vi "RL Connect.vi"() -> ()   [LabVIEW 2019]
uses:
  C:/Users/wego/Documents/GitHub/Ycar/LabVIEW/Gmap/dll/GMap.NET.WindowsForms.dll
  Gmap/dll/GMap.NET.WindowsForms.dll
  Ctrl/ublox-ui_main.ctl
  Ctrl/gnss_config-2.ctl
  Ctrl/Ntrip_Account_db.ctl
  Ctrl/Ntrip error-leds.ctl
  Ctrl/cmd_common.ctl
  Ctrl/cmd_ini-add-read.ctl
  Ctrl/cmd_ini-RW.ctl
  Ctrl/GNSS-Ntrip ref.ctl
  Gmap/gmap_fgv-cmd.ctl
  Ctrl/GNSS-Ntrip config.ctl
  Ctrl/error_state-val.ctl
panel:
  out "Version String":string
  in  "Ntrip connect":bool
  out "status":T1={"GNSS Serial"=0, "NMEA val"=0, "Send Serial"=0, "Ntrip TCP"=0, "RTCM val"=0, "GMAP"=0, "TBD1"=2, "TBD2"=2, "TBD3"=2}
  in  "Send-Serial Start-Stop":bool
  in  "GNSS Start-Stop":bool
  in  "stop":bool
  in  "gmap center":bool
  in  "Gmap Lon":dbl format="%.7f"
  in  "Gmap Lat":dbl format="%.7f"
  in  "GMapControl":refnum<k24>(container)
  out "GNSS time":string
  out "Ntrip conn":bool
  out "NMEA val":bool
  in  "main tap":T2(tab)
  out "TM\nptn":u32(slide) scale=0.0..200.0
  out "Sea Level":dbl
  out "N of Satellites":i32
  out "TM graph":T3(graph)=[{"TM array"=[{"Y(E)"=195478.83340938148, "X(N)"=532749.6315443226}, {"Y(E)"=195478.83340938148, "X(N)"=532749.6315443226}, {"Y(E)"=195478.83340938148, "X(N)"=532749.6315443226}, {"Y(E)"=195478.83340938148, "X(N)"=532749.6315443226}, {"Y(E)"=195478.83340938148, "X(N)"=532749.6315443226}, {"Y(E)"=195478.83340938148, "X(N)"=532749.6315443226}, {"Y(E)"=195478.83340938148, "X(N)"=532749.6315443226}, {"Y(E)"=195478.83340938148, "X(N)"=532749.6315443226}, {"Y(E)"=195478.83340938148, "X(N)"=532749.6315443226}, {"Y(E)"=195478.83340938148, "X(N)"=532749.6315443226}, {"Y(E)"=195478.80387262133, "X(N)"=532749.5945652778}, {"Y(E)"=195478.80387262133, "X(N)"=532749.5945652778}, {"Y(E)"=195478.80387262133, "X(N)"=532749.5945652778}, {"Y(E)"=195478.80387262133, "X(N)"=532749.5945652778}, {"Y(E)"=195478.80387262133, "X(N)"=532749.5945652778}, {"Y(E)"=195478.80387262133, "X(N)"=532749.5945652778}, {"Y(E)"=195478.80387262133, "X(N)"=532749.5945652778}, {"Y(E)"=195478.80387262133, "X(N)"=532749.5945652778}, {"Y(E)"=195478.80387262133, "X(N)"=532749.5945652778}, {"Y(E)"=195478.80387262133, "X(N)"=532749.5945652778}, {"Y(E)"=195478.80387262133, "X(N)"=532749.5945652778}, {"Y(E)"=195478.80387262133, "X(N)"=532749.5945652778}, {"Y(E)"=195478.80387262133, "X(N)"=532749.5945652778}, {"Y(E)"=195478.86283602339, "X(N)"=532749.4650507653}, {"Y(E)"=195478.86283602339, "X(N)"=532749.4650507653}, {"Y(E)"=195478.86283602339, "X(N)"=532749.4650507653}, {"Y(E)"=195478.86283602339, "X(N)"=532749.4650507653}, {"Y(E)"=195478.86283602339, "X(N)"=532749.4650507653}, {"Y(E)"=195478.86283602339, "X(N)"=532749.4650507653}, {"Y(E)"=195478.86283602339, "X(N)"=532749.4650507653}, {"Y(E)"=195478.86283602339, "X(N)"=532749.4650507653}, {"Y(E)"=195478.86283602339, "X(N)"=532749.4650507653}, {"Y(E)"=195478.86283602339, "X(N)"=532749.4650507653}, {"Y(E)"=195478.86283602339, "X(N)"=532749.4650507653}, {"Y(E)"=195478.86283602339, "X(N)"=532749.4650507653}, {"Y(E)"=195478.86283602339, "X(N)"=532749.4650507653}, {"Y(E)"=195478.8185809412, "X(N)"=532749.5020697443}, {"Y(E)"=195478.8185809412, "X(N)"=532749.5020697443}, {"Y(E)"=195478.8185809412, "X(N)"=532749.5020697443}, {"Y(E)"=195478.8185809412, "X(N)"=532749.5020697443}, {"Y(E)"=195478.8185809412, "X(N)"=532749.5020697443}, {"Y(E)"=195478.8185809412, "X(N)"=532749.5020697443}, {"Y(E)"=195478.8185809412, "X(N)"=532749.5020697443}, {"Y(E)"=195478.8185809412, "X(N)"=532749.5020697443}, {"Y(E)"=195478.8185809412, "X(N)"=532749.5020697443}, {"Y(E)"=195478.8185809412, "X(N)"=532749.5020697443}, {"Y(E)"=195478.8185809412, "X(N)"=532749.5020697443}, {"Y(E)"=195478.8185809412, "X(N)"=532749.5020697443}, {"Y(E)"=195478.8185809412, "X(N)"=532749.5020697443}, {"Y(E)"=195478.8333493192, "X(N)"=532749.5205592669}, {"Y(E)"=195478.8333493192, "X(N)"=532749.5205592669}, {"Y(E)"=195478.8333493192, "X(N)"=532749.5205592669}, {"Y(E)"=195478.8333493192, "X(N)"=532749.5205592669}, {"Y(E)"=195478.8333493192, "X(N)"=532749.5205592669}, {"Y(E)"=195478.8333493192, "X(N)"=532749.5205592669}, {"Y(E)"=195478.8333493192, "X(N)"=532749.5205592669}, {"Y(E)"=195478.8333493192, "X(N)"=532749.5205592669}, {"Y(E)"=195478.8333493192, "X(N)"=532749.5205592669}, {"Y(E)"=195478.8333493192, "X(N)"=532749.5205592669}, {"Y(E)"=195478.8333493192, "X(N)"=532749.5205592669}, {"Y(E)"=195478.8333493192, "X(N)"=532749.5205592669}, {"Y(E)"=195478.81854089958, "X(N)"=532749.4280797082}, {"Y(E)"=195478.81854089958, "X(N)"=532749.4280797082}, {"Y(E)"=195478.81854089958, "X(N)"=532749.4280797082}, {"Y(E)"=195478.81854089958, "X(N)"=532749.4280797082}, {"Y(E)"=195478.81854089958, "X(N)"=532749.4280797082}, {"Y(E)"=195478.81854089958, "X(N)"=532749.4280797082}, {"Y(E)"=195478.81854089958, "X(N)"=532749.4280797082}, {"Y(E)"=195478.81854089958, "X(N)"=532749.4280797082}, {"Y(E)"=195478.81854089958, "X(N)"=532749.4280797082}, {"Y(E)"=195478.81854089958, "X(N)"=532749.4280797082}, {"Y(E)"=195478.81854089958, "X(N)"=532749.4280797082}, {"Y(E)"=195478.81854089958, "X(N)"=532749.4280797082}, {"Y(E)"=195478.81854089958, "X(N)"=532749.4280797082}, {"Y(E)"=195478.8332592258, "X(N)"=532749.3540816847}, {"Y(E)"=195478.8332592258, "X(N)"=532749.3540816847}, {"Y(E)"=195478.8332592258, "X(N)"=532749.3540816847}, {"Y(E)"=195478.8332592258, "X(N)"=532749.3540816847}, {"Y(E)"=195478.8332592258, "X(N)"=532749.3540816847}, {"Y(E)"=195478.8332592258, "X(N)"=532749.3540816847}, {"Y(E)"=195478.8332592258, "X(N)"=532749.3540816847}, {"Y(E)"=195478.8332592258, "X(N)"=532749.3540816847}, {"Y(E)"=195478.8332592258, "X(N)"=532749.3540816847}, {"Y(E)"=195478.8332592258, "X(N)"=532749.3540816847}, {"Y(E)"=195478.8332592258, "X(N)"=532749.3540816847}, {"Y(E)"=195478.8332592258, "X(N)"=532749.3540816847}, {"Y(E)"=195478.8332592258, "X(N)"=532749.3540816847}, {"Y(E)"=195478.61200383154, "X(N)"=532749.5761715989}, {"Y(E)"=195478.61200383154, "X(N)"=532749.5761715989}, {"Y(E)"=195478.61200383154, "X(N)"=532749.5761715989}, {"Y(E)"=195478.61200383154, "X(N)"=532749.5761715989}, {"Y(E)"=195478.61200383154, "X(N)"=532749.5761715989}, {"Y(E)"=195478.61200383154, "X(N)"=532749.5761715989}, {"Y(E)"=195478.61200383154, "X(N)"=532749.5761715989}, {"Y(E)"=195478.61200383154, "X(N)"=532749.5761715989}, {"Y(E)"=195478.61200383154, "X(N)"=532749.5761715989}, {"Y(E)"=195478.61200383154, "X(N)"=532749.5761715989}, {"Y(E)"=195478.61200383154, "X(N)"=532749.5761715989}, {"Y(E)"=195478.61200383154, "X(N)"=532749.5761715989}, {"Y(E)"=195478.61200383154, "X(N)"=532749.5761715989}, {"Y(E)"=195478.61197379892, "X(N)"=532749.5206790727}, {"Y(E)"=195478.61197379892, "X(N)"=532749.5206790727}, {"Y(E)"=195478.61197379892, "X(N)"=532749.5206790727}, {"Y(E)"=195478.61197379892, "X(N)"=532749.5206790727}, {"Y(E)"=195478.61197379892, "X(N)"=532749.5206790727}, {"Y(E)"=195478.61197379892, "X(N)"=532749.5206790727}, {"Y(E)"=195478.61197379892, "X(N)"=532749.5206790727}, {"Y(E)"=195478.61197379892, "X(N)"=532749.5206790727}, {"Y(E)"=195478.61197379892, "X(N)"=532749.5206790727}, {"Y(E)"=195478.61197379892, "X(N)"=532749.5206790727}, {"Y(E)"=195478.61197379892, "X(N)"=532749.5206790727}, {"Y(E)"=195478.61197379892, "X(N)"=532749.5206790727}, {"Y(E)"=195478.61197379892, "X(N)"=532749.5206790727}, {"Y(E)"=195478.64144048005, "X(N)"=532749.4281755526}, {"Y(E)"=195478.64144048005, "X(N)"=532749.4281755526}, {"Y(E)"=195478.64144048005, "X(N)"=532749.4281755526}, {"Y(E)"=195478.64144048005, "X(N)"=532749.4281755526}, {"Y(E)"=195478.64144048005, "X(N)"=532749.4281755526}, {"Y(E)"=195478.64144048005, "X(N)"=532749.4281755526}, {"Y(E)"=195478.64144048005, "X(N)"=532749.4281755526}, {"Y(E)"=195478.64144048005, "X(N)"=532749.4281755526}, {"Y(E)"=195478.64144048005, "X(N)"=532749.4281755526}, {"Y(E)"=195478.64144048005, "X(N)"=532749.4281755526}, {"Y(E)"=195478.64144048005, "X(N)"=532749.4281755526}, {"Y(E)"=195478.64144048005, "X(N)"=532749.4281755526}, {"Y(E)"=195478.64144048005, "X(N)"=532749.4281755526}, {"Y(E)"=195478.56754852948, "X(N)"=532749.2432403986}, {"Y(E)"=195478.56754852948, "X(N)"=532749.2432403986}, {"Y(E)"=195478.56754852948, "X(N)"=532749.2432403986}, {"Y(E)"=195478.56754852948, "X(N)"=532749.2432403986}, {"Y(E)"=195478.56754852948, "X(N)"=532749.2432403986}, {"Y(E)"=195478.56754852948, "X(N)"=532749.2432403986}, {"Y(E)"=195478.56754852948, "X(N)"=532749.2432403986}, {"Y(E)"=195478.56754852948, "X(N)"=532749.2432403986}, {"Y(E)"=195478.56754852948, "X(N)"=532749.2432403986}, {"Y(E)"=195478.56754852948, "X(N)"=532749.2432403986}, {"Y(E)"=195478.56754852948, "X(N)"=532749.2432403986}, {"Y(E)"=195478.56754852948, "X(N)"=532749.2432403986}, {"Y(E)"=195478.56754852948, "X(N)"=532749.2432403986}, {"Y(E)"=195478.5822568451, "X(N)"=532749.1507448669}, {"Y(E)"=195478.5822568451, "X(N)"=532749.1507448669}, {"Y(E)"=195478.5822568451, "X(N)"=532749.1507448669}, {"Y(E)"=195478.5822568451, "X(N)"=532749.1507448669}, {"Y(E)"=195478.5822568451, "X(N)"=532749.1507448669}, {"Y(E)"=195478.5822568451, "X(N)"=532749.1507448669}, {"Y(E)"=195478.5822568451, "X(N)"=532749.1507448669}, {"Y(E)"=195478.5822568451, "X(N)"=532749.1507448669}, {"Y(E)"=195478.5822568451, "X(N)"=532749.1507448669}, {"Y(E)"=195478.5822568451, "X(N)"=532749.1507448669}, {"Y(E)"=195478.5822568451, "X(N)"=532749.1507448669}, {"Y(E)"=195478.5822568451, "X(N)"=532749.1507448669}, {"Y(E)"=195478.5822568451, "X(N)"=532749.1507448669}, {"Y(E)"=195478.3755095352, "X(N)"=532748.9103890732}, {"Y(E)"=195478.3755095352, "X(N)"=532748.9103890732}, {"Y(E)"=195478.3755095352, "X(N)"=532748.9103890732}, {"Y(E)"=195478.3755095352, "X(N)"=532748.9103890732}, {"Y(E)"=195478.3755095352, "X(N)"=532748.9103890732}, {"Y(E)"=195478.3755095352, "X(N)"=532748.9103890732}, {"Y(E)"=195478.3755095352, "X(N)"=532748.9103890732}, {"Y(E)"=195478.3755095352, "X(N)"=532748.9103890732}, {"Y(E)"=195478.3755095352, "X(N)"=532748.9103890732}, {"Y(E)"=195478.3755095352, "X(N)"=532748.9103890732}, {"Y(E)"=195478.3755095352, "X(N)"=532748.9103890732}, {"Y(E)"=195478.3755095352, "X(N)"=532748.9103890732}, {"Y(E)"=195478.3755095352, "X(N)"=532748.9103890732}, {"Y(E)"=195478.37543945547, "X(N)"=532748.78090651}, {"Y(E)"=195478.37543945547, "X(N)"=532748.78090651}, {"Y(E)"=195478.37543945547, "X(N)"=532748.78090651}, {"Y(E)"=195478.37543945547, "X(N)"=532748.78090651}, {"Y(E)"=195478.37543945547, "X(N)"=532748.78090651}, {"Y(E)"=195478.37543945547, "X(N)"=532748.78090651}, {"Y(E)"=195478.37543945547, "X(N)"=532748.78090651}, {"Y(E)"=195478.37543945547, "X(N)"=532748.78090651}, {"Y(E)"=195478.37543945547, "X(N)"=532748.78090651}, {"Y(E)"=195478.37543945547, "X(N)"=532748.78090651}, {"Y(E)"=195478.37543945547, "X(N)"=532748.78090651}, {"Y(E)"=195478.37543945547, "X(N)"=532748.78090651}, {"Y(E)"=195478.5082848043, "X(N)"=532748.8178296402}, {"Y(E)"=195478.5082848043, "X(N)"=532748.8178296402}, {"Y(E)"=195478.5082848043, "X(N)"=532748.8178296402}, {"Y(E)"=195478.5082848043, "X(N)"=532748.8178296402}, {"Y(E)"=195478.5082848043, "X(N)"=532748.8178296402}, {"Y(E)"=195478.5082848043, "X(N)"=532748.8178296402}, {"Y(E)"=195478.5082848043, "X(N)"=532748.8178296402}, {"Y(E)"=195478.5082848043, "X(N)"=532748.8178296402}, {"Y(E)"=195478.5082848043, "X(N)"=532748.8178296402}, {"Y(E)"=195478.5082848043, "X(N)"=532748.8178296402}, {"Y(E)"=195478.5082848043, "X(N)"=532748.8178296402}, {"Y(E)"=195478.5082848043, "X(N)"=532748.8178296402}, {"Y(E)"=195478.5082848043, "X(N)"=532748.8178296402}, {"Y(E)"=195478.7001636224, "X(N)"=532748.8547208244}, {"Y(E)"=195478.7001636224, "X(N)"=532748.8547208244}, {"Y(E)"=195478.7001636224, "X(N)"=532748.8547208244}, {"Y(E)"=195478.7001636224, "X(N)"=532748.8547208244}, {"Y(E)"=195478.7001636224, "X(N)"=532748.8547208244}, {"Y(E)"=195478.7001636224, "X(N)"=532748.8547208244}, {"Y(E)"=195478.7001636224, "X(N)"=532748.8547208244}, {"Y(E)"=195478.7001636224, "X(N)"=532748.8547208244}, {"Y(E)"=195478.7001636224, "X(N)"=532748.8547208244}, {"Y(E)"=195478.7001636224, "X(N)"=532748.8547208244}]}, {"TM array"=[{"Y(E)"=195478.60442441847, "X(N)"=532749.6892681528}, {"Y(E)"=195478.63475492285, "X(N)"=532749.6883149784}, {"Y(E)"=195478.6649657266, "X(N)"=532749.6854592166}, {"Y(E)"=195478.69493760145, "X(N)"=532749.680712138}, {"Y(E)"=195478.72455226214, "X(N)"=532749.6740924771}, {"Y(E)"=195478.7536928331, "X(N)"=532749.6656263586}, {"Y(E)"=195478.7822443098, "X(N)"=532749.6553471944}, {"Y(E)"=195478.81009401265, "X(N)"=532749.6432955518}, {"Y(E)"=195478.83713203156, "X(N)"=532749.6295189931}, {"Y(E)"=195478.86325165984, "X(N)"=532749.6140718879}, {"Y(E)"=195478.88834981524, "X(N)"=532749.5970151991}, {"Y(E)"=195478.91232744683, "X(N)"=532749.5784162417}, {"Y(E)"=195478.93508992583, "X(N)"=532749.5583484169}, {"Y(E)"=195478.95654741913, "X(N)"=532749.5368909236}, {"Y(E)"=195478.97661524382, "X(N)"=532749.5141284446}, {"Y(E)"=195478.99521420136, "X(N)"=532749.490150813}, {"Y(E)"=195479.01227089018, "X(N)"=532749.4650526576}, {"Y(E)"=195479.02771799528, "X(N)"=532749.4389330294}, {"Y(E)"=195479.04149455403, "X(N)"=532749.4118950105}, {"Y(E)"=195479.0535461966, "X(N)"=532749.3840453076}, {"Y(E)"=195479.06382536073, "X(N)"=532749.3554938309}, {"Y(E)"=195479.0722914792, "X(N)"=532749.32635326}, {"Y(E)"=195479.07891114015, "X(N)"=532749.2967385993}, {"Y(E)"=195479.0836582188, "X(N)"=532749.2667667244}, {"Y(E)"=195479.08651398055, "X(N)"=532749.2365559207}, {"Y(E)"=195479.08746715504, "X(N)"=532749.2062254163}, {"Y(E)"=195479.08651398055, "X(N)"=532749.1758949119}, {"Y(E)"=195479.0836582188, "X(N)"=532749.1456841081}, {"Y(E)"=195479.07891114015, "X(N)"=532749.1157122332}, {"Y(E)"=195479.0722914792, "X(N)"=532749.0860975726}, {"Y(E)"=195479.06382536073, "X(N)"=532749.0569570017}, {"Y(E)"=195479.0535461966, "X(N)"=532749.0284055249}, {"Y(E)"=195479.04149455403, "X(N)"=532749.000555822}, {"Y(E)"=195479.02771799528, "X(N)"=532748.9735178031}, {"Y(E)"=195479.01227089018, "X(N)"=532748.9473981749}, {"Y(E)"=195478.99521420136, "X(N)"=532748.9223000195}, {"Y(E)"=195478.97661524382, "X(N)"=532748.898322388}, {"Y(E)"=195478.95654741913, "X(N)"=532748.8755599089}, {"Y(E)"=195478.93508992583, "X(N)"=532748.8541024156}, {"Y(E)"=195478.91232744683, "X(N)"=532748.8340345909}, {"Y(E)"=195478.88834981524, "X(N)"=532748.8154356334}, {"Y(E)"=195478.86325165984, "X(N)"=532748.7983789446}, {"Y(E)"=195478.83713203156, "X(N)"=532748.7829318395}, {"Y(E)"=195478.81009401265, "X(N)"=532748.7691552808}, {"Y(E)"=195478.7822443098, "X(N)"=532748.7571036381}, {"Y(E)"=195478.7536928331, "X(N)"=532748.746824474}, {"Y(E)"=195478.72455226214, "X(N)"=532748.7383583555}, {"Y(E)"=195478.69493760145, "X(N)"=532748.7317386946}, {"Y(E)"=195478.6649657266, "X(N)"=532748.726991616}, {"Y(E)"=195478.63475492285, "X(N)"=532748.7241358542}, {"Y(E)"=195478.60442441847, "X(N)"=532748.7231826797}, {"Y(E)"=195478.5740939141, "X(N)"=532748.7241358542}, {"Y(E)"=195478.54388311034, "X(N)"=532748.726991616}, {"Y(E)"=195478.5139112355, "X(N)"=532748.7317386946}, {"Y(E)"=195478.4842965748, "X(N)"=532748.7383583555}, {"Y(E)"=195478.45515600385, "X(N)"=532748.746824474}, {"Y(E)"=195478.42660452714, "X(N)"=532748.7571036381}, {"Y(E)"=195478.3987548243, "X(N)"=532748.7691552808}, {"Y(E)"=195478.37171680538, "X(N)"=532748.7829318395}, {"Y(E)"=195478.3455971771, "X(N)"=532748.7983789446}, {"Y(E)"=195478.3204990217, "X(N)"=532748.8154356334}, {"Y(E)"=195478.29652139012, "X(N)"=532748.8340345909}, {"Y(E)"=195478.27375891112, "X(N)"=532748.8541024156}, {"Y(E)"=195478.25230141782, "X(N)"=532748.8755599089}, {"Y(E)"=195478.23223359312, "X(N)"=532748.898322388}, {"Y(E)"=195478.21363463558, "X(N)"=532748.9223000195}, {"Y(E)"=195478.19657794677, "X(N)"=532748.9473981749}, {"Y(E)"=195478.18113084167, "X(N)"=532748.9735178031}, {"Y(E)"=195478.16735428292, "X(N)"=532749.000555822}, {"Y(E)"=195478.15530264034, "X(N)"=532749.0284055249}, {"Y(E)"=195478.14502347622, "X(N)"=532749.0569570017}, {"Y(E)"=195478.13655735774, "X(N)"=532749.0860975726}, {"Y(E)"=195478.1299376968, "X(N)"=532749.1157122332}, {"Y(E)"=195478.12519061816, "X(N)"=532749.1456841081}, {"Y(E)"=195478.1223348564, "X(N)"=532749.1758949119}, {"Y(E)"=195478.1213816819, "X(N)"=532749.2062254163}, {"Y(E)"=195478.1223348564, "X(N)"=532749.2365559207}, {"Y(E)"=195478.12519061816, "X(N)"=532749.2667667244}, {"Y(E)"=195478.1299376968, "X(N)"=532749.2967385993}, {"Y(E)"=195478.13655735774, "X(N)"=532749.32635326}, {"Y(E)"=195478.14502347622, "X(N)"=532749.3554938309}, {"Y(E)"=195478.15530264034, "X(N)"=532749.3840453076}, {"Y(E)"=195478.16735428292, "X(N)"=532749.4118950105}, {"Y(E)"=195478.18113084167, "X(N)"=532749.4389330294}, {"Y(E)"=195478.19657794677, "X(N)"=532749.4650526576}, {"Y(E)"=195478.21363463558, "X(N)"=532749.490150813}, {"Y(E)"=195478.23223359312, "X(N)"=532749.5141284446}, {"Y(E)"=195478.25230141782, "X(N)"=532749.5368909236}, {"Y(E)"=195478.27375891112, "X(N)"=532749.5583484169}, {"Y(E)"=195478.29652139012, "X(N)"=532749.5784162417}, {"Y(E)"=195478.3204990217, "X(N)"=532749.5970151991}, {"Y(E)"=195478.3455971771, "X(N)"=532749.6140718879}, {"Y(E)"=195478.37171680538, "X(N)"=532749.6295189931}, {"Y(E)"=195478.3987548243, "X(N)"=532749.6432955518}, {"Y(E)"=195478.42660452714, "X(N)"=532749.6553471944}, {"Y(E)"=195478.45515600385, "X(N)"=532749.6656263586}, {"Y(E)"=195478.4842965748, "X(N)"=532749.6740924771}, {"Y(E)"=195478.5139112355, "X(N)"=532749.680712138}, {"Y(E)"=195478.54388311034, "X(N)"=532749.6854592166}, {"Y(E)"=195478.5740939141, "X(N)"=532749.6883149784}, {"Y(E)"=195478.60442441847, "X(N)"=532749.6892681528}]}, {"TM array"=[{"Y(E)"=195478.60442441847, "X(N)"=532750.2062254163}, {"Y(E)"=195478.667214938, "X(N)"=532750.2042521447}, {"Y(E)"=195478.72975765204, "X(N)"=532750.1983401176}, {"Y(E)"=195478.79180573305, "X(N)"=532750.188512667}, {"Y(E)"=195478.85311430565, "X(N)"=532750.1748085774}, {"Y(E)"=195478.91344141285, "X(N)"=532750.1572819325}, {"Y(E)"=195478.97254897116, "X(N)"=532750.1360019022}, {"Y(E)"=195479.03020371005, "X(N)"=532750.1110524688}, {"Y(E)"=195479.08617809258, "X(N)"=532750.0825320963}, {"Y(E)"=195479.14025121345, "X(N)"=532750.0505533417}, {"Y(E)"=195479.19220967076, "X(N)"=532750.0152424106}, {"Y(E)"=195479.24184840822, "X(N)"=532749.9767386591}, {"Y(E)"=195479.2889715244, "X(N)"=532749.9351940437}, {"Y(E)"=195479.3333930459, "X(N)"=532749.8907725222}, {"Y(E)"=195479.37493766125, "X(N)"=532749.843649406}, {"Y(E)"=195479.41344141285, "X(N)"=532749.7940106685}, {"Y(E)"=195479.44875234397, "X(N)"=532749.7420522113}, {"Y(E)"=195479.4807310985, "X(N)"=532749.6879790904}, {"Y(E)"=195479.50925147094, "X(N)"=532749.6320047078}, {"Y(E)"=195479.53420090437, "X(N)"=532749.5743499689}, {"Y(E)"=195479.55548093477, "X(N)"=532749.5152424106}, {"Y(E)"=195479.5730075796, "X(N)"=532749.4549153034}, {"Y(E)"=195479.5867116692, "X(N)"=532749.3936067309}, {"Y(E)"=195479.59653911978, "X(N)"=532749.3315586499}, {"Y(E)"=195479.6024511469, "X(N)"=532749.2690159358}, {"Y(E)"=195479.60442441847, "X(N)"=532749.2062254163}, {"Y(E)"=195479.6024511469, "X(N)"=532749.1434348967}, {"Y(E)"=195479.59653911978, "X(N)"=532749.0808921827}, {"Y(E)"=195479.5867116692, "X(N)"=532749.0188441017}, {"Y(E)"=195479.5730075796, "X(N)"=532748.9575355292}, {"Y(E)"=195479.55548093477, "X(N)"=532748.897208422}, {"Y(E)"=195479.53420090437, "X(N)"=532748.8381008636}, {"Y(E)"=195479.50925147094, "X(N)"=532748.7804461247}, {"Y(E)"=195479.4807310985, "X(N)"=532748.7244717422}, {"Y(E)"=195479.44875234397, "X(N)"=532748.6703986212}, {"Y(E)"=195479.41344141285, "X(N)"=532748.618440164}, {"Y(E)"=195479.37493766125, "X(N)"=532748.5688014266}, {"Y(E)"=195479.3333930459, "X(N)"=532748.5216783104}, {"Y(E)"=195479.2889715244, "X(N)"=532748.4772567889}, {"Y(E)"=195479.24184840822, "X(N)"=532748.4357121735}, {"Y(E)"=195479.19220967076, "X(N)"=532748.397208422}, {"Y(E)"=195479.14025121345, "X(N)"=532748.3618974908}, {"Y(E)"=195479.08617809258, "X(N)"=532748.3299187362}, {"Y(E)"=195479.03020371005, "X(N)"=532748.3013983638}, {"Y(E)"=195478.97254897116, "X(N)"=532748.2764489304}, {"Y(E)"=195478.91344141285, "X(N)"=532748.2551689}, {"Y(E)"=195478.85311430565, "X(N)"=532748.2376422551}, {"Y(E)"=195478.79180573305, "X(N)"=532748.2239381656}, {"Y(E)"=195478.72975765204, "X(N)"=532748.214110715}, {"Y(E)"=195478.667214938, "X(N)"=532748.2081986879}, {"Y(E)"=195478.60442441847, "X(N)"=532748.2062254163}, {"Y(E)"=195478.54163389895, "X(N)"=532748.2081986879}, {"Y(E)"=195478.4790911849, "X(N)"=532748.214110715}, {"Y(E)"=195478.4170431039, "X(N)"=532748.2239381656}, {"Y(E)"=195478.3557345313, "X(N)"=532748.2376422551}, {"Y(E)"=195478.2954074241, "X(N)"=532748.2551689}, {"Y(E)"=195478.2362998658, "X(N)"=532748.2764489304}, {"Y(E)"=195478.1786451269, "X(N)"=532748.3013983638}, {"Y(E)"=195478.12267074437, "X(N)"=532748.3299187362}, {"Y(E)"=195478.0685976235, "X(N)"=532748.3618974908}, {"Y(E)"=195478.0166391662, "X(N)"=532748.397208422}, {"Y(E)"=195477.96700042873, "X(N)"=532748.4357121735}, {"Y(E)"=195477.91987731255, "X(N)"=532748.4772567889}, {"Y(E)"=195477.87545579104, "X(N)"=532748.5216783104}, {"Y(E)"=195477.8339111757, "X(N)"=532748.5688014266}, {"Y(E)"=195477.7954074241, "X(N)"=532748.618440164}, {"Y(E)"=195477.76009649297, "X(N)"=532748.6703986212}, {"Y(E)"=195477.72811773844, "X(N)"=532748.7244717422}, {"Y(E)"=195477.699597366, "X(N)"=532748.7804461247}, {"Y(E)"=195477.67464793258, "X(N)"=532748.8381008636}, {"Y(E)"=195477.65336790218, "X(N)"=532748.897208422}, {"Y(E)"=195477.63584125735, "X(N)"=532748.9575355292}, {"Y(E)"=195477.62213716775, "X(N)"=532749.0188441017}, {"Y(E)"=195477.61230971717, "X(N)"=532749.0808921827}, {"Y(E)"=195477.60639769005, "X(N)"=532749.1434348967}, {"Y(E)"=195477.60442441847, "X(N)"=532749.2062254163}, {"Y(E)"=195477.60639769005, "X(N)"=532749.2690159358}, {"Y(E)"=195477.61230971717, "X(N)"=532749.3315586499}, {"Y(E)"=195477.62213716775, "X(N)"=532749.3936067309}, {"Y(E)"=195477.63584125735, "X(N)"=532749.4549153034}, {"Y(E)"=195477.65336790218, "X(N)"=532749.5152424106}, {"Y(E)"=195477.67464793258, "X(N)"=532749.5743499689}, {"Y(E)"=195477.699597366, "X(N)"=532749.6320047078}, {"Y(E)"=195477.72811773844, "X(N)"=532749.6879790904}, {"Y(E)"=195477.76009649297, "X(N)"=532749.7420522113}, {"Y(E)"=195477.7954074241, "X(N)"=532749.7940106685}, {"Y(E)"=195477.8339111757, "X(N)"=532749.843649406}, {"Y(E)"=195477.87545579104, "X(N)"=532749.8907725222}, {"Y(E)"=195477.91987731255, "X(N)"=532749.9351940437}, {"Y(E)"=195477.96700042873, "X(N)"=532749.9767386591}, {"Y(E)"=195478.0166391662, "X(N)"=532750.0152424106}, {"Y(E)"=195478.0685976235, "X(N)"=532750.0505533417}, {"Y(E)"=195478.12267074437, "X(N)"=532750.0825320963}, {"Y(E)"=195478.1786451269, "X(N)"=532750.1110524688}, {"Y(E)"=195478.2362998658, "X(N)"=532750.1360019022}, {"Y(E)"=195478.2954074241, "X(N)"=532750.1572819325}, {"Y(E)"=195478.3557345313, "X(N)"=532750.1748085774}, {"Y(E)"=195478.4170431039, "X(N)"=532750.188512667}, {"Y(E)"=195478.4790911849, "X(N)"=532750.1983401176}, {"Y(E)"=195478.54163389895, "X(N)"=532750.2042521447}, {"Y(E)"=195478.60442441847, "X(N)"=532750.2062254163}]}, {"TM array"=[{"Y(E)"=195478.60442441847, "X(N)"=532751.2062254163}, {"Y(E)"=195478.73000545753, "X(N)"=532751.2022788732}, {"Y(E)"=195478.8550908856, "X(N)"=532751.1904548189}, {"Y(E)"=195478.97918704763, "X(N)"=532751.1707999178}, {"Y(E)"=195479.10180419282, "X(N)"=532751.1433917385}, {"Y(E)"=195479.22245840722, "X(N)"=532751.1083384489}, {"Y(E)"=195479.34067352384, "X(N)"=532751.0657783881}, {"Y(E)"=195479.4559830016, "X(N)"=532751.0158795213}, {"Y(E)"=195479.56793176668, "X(N)"=532750.9588387763}, {"Y(E)"=195479.67607800843, "X(N)"=532750.8948812673}, {"Y(E)"=195479.77999492307, "X(N)"=532750.824259405}, {"Y(E)"=195479.879272398, "X(N)"=532750.7472519018}, {"Y(E)"=195479.97351863034, "X(N)"=532750.6641626711}, {"Y(E)"=195480.0623616733, "X(N)"=532750.5753196281}, {"Y(E)"=195480.14545090403, "X(N)"=532750.4810733958}, {"Y(E)"=195480.22245840722, "X(N)"=532750.3817959209}, {"Y(E)"=195480.29308026948, "X(N)"=532750.2778790062}, {"Y(E)"=195480.35703777857, "X(N)"=532750.1697327645}, {"Y(E)"=195480.4140785234, "X(N)"=532750.0577839994}, {"Y(E)"=195480.46397739026, "X(N)"=532749.9424745217}, {"Y(E)"=195480.50653745106, "X(N)"=532749.824259405}, {"Y(E)"=195480.54159074073, "X(N)"=532749.7036051906}, {"Y(E)"=195480.56899891995, "X(N)"=532749.5809880454}, {"Y(E)"=195480.5886538211, "X(N)"=532749.4568918834}, {"Y(E)"=195480.60047787533, "X(N)"=532749.3318064554}, {"Y(E)"=195480.60442441847, "X(N)"=532749.2062254163}, {"Y(E)"=195480.60047787533, "X(N)"=532749.0806443772}, {"Y(E)"=195480.5886538211, "X(N)"=532748.9555589492}, {"Y(E)"=195480.56899891995, "X(N)"=532748.8314627871}, {"Y(E)"=195480.54159074073, "X(N)"=532748.7088456419}, {"Y(E)"=195480.50653745106, "X(N)"=532748.5881914275}, {"Y(E)"=195480.46397739026, "X(N)"=532748.4699763109}, {"Y(E)"=195480.4140785234, "X(N)"=532748.3546668332}, {"Y(E)"=195480.35703777857, "X(N)"=532748.2427180681}, {"Y(E)"=195480.29308026948, "X(N)"=532748.1345718263}, {"Y(E)"=195480.22245840722, "X(N)"=532748.0306549117}, {"Y(E)"=195480.14545090403, "X(N)"=532747.9313774367}, {"Y(E)"=195480.0623616733, "X(N)"=532747.8371312044}, {"Y(E)"=195479.97351863034, "X(N)"=532747.7482881615}, {"Y(E)"=195479.879272398, "X(N)"=532747.6651989308}, {"Y(E)"=195479.77999492307, "X(N)"=532747.5881914275}, {"Y(E)"=195479.67607800843, "X(N)"=532747.5175695652}, {"Y(E)"=195479.56793176668, "X(N)"=532747.4536120562}, {"Y(E)"=195479.4559830016, "X(N)"=532747.3965713113}, {"Y(E)"=195479.34067352384, "X(N)"=532747.3466724445}, {"Y(E)"=195479.22245840722, "X(N)"=532747.3041123836}, {"Y(E)"=195479.10180419282, "X(N)"=532747.269059094}, {"Y(E)"=195478.97918704763, "X(N)"=532747.2416509148}, {"Y(E)"=195478.8550908856, "X(N)"=532747.2219960137}, {"Y(E)"=195478.73000545753, "X(N)"=532747.2101719594}, {"Y(E)"=195478.60442441847, "X(N)"=532747.2062254163}, {"Y(E)"=195478.47884337942, "X(N)"=532747.2101719594}, {"Y(E)"=195478.35375795135, "X(N)"=532747.2219960137}, {"Y(E)"=195478.22966178932, "X(N)"=532747.2416509148}, {"Y(E)"=195478.10704464413, "X(N)"=532747.269059094}, {"Y(E)"=195477.98639042972, "X(N)"=532747.3041123836}, {"Y(E)"=195477.8681753131, "X(N)"=532747.3466724445}, {"Y(E)"=195477.75286583535, "X(N)"=532747.3965713113}, {"Y(E)"=195477.64091707027, "X(N)"=532747.4536120562}, {"Y(E)"=195477.53277082852, "X(N)"=532747.5175695652}, {"Y(E)"=195477.42885391388, "X(N)"=532747.5881914275}, {"Y(E)"=195477.32957643896, "X(N)"=532747.6651989308}, {"Y(E)"=195477.2353302066, "X(N)"=532747.7482881615}, {"Y(E)"=195477.14648716364, "X(N)"=532747.8371312044}, {"Y(E)"=195477.0633979329, "X(N)"=532747.9313774367}, {"Y(E)"=195476.98639042972, "X(N)"=532748.0306549117}, {"Y(E)"=195476.91576856747, "X(N)"=532748.1345718263}, {"Y(E)"=195476.85181105838, "X(N)"=532748.2427180681}, {"Y(E)"=195476.79477031354, "X(N)"=532748.3546668332}, {"Y(E)"=195476.7448714467, "X(N)"=532748.4699763109}, {"Y(E)"=195476.7023113859, "X(N)"=532748.5881914275}, {"Y(E)"=195476.66725809622, "X(N)"=532748.7088456419}, {"Y(E)"=195476.639849917, "X(N)"=532748.8314627871}, {"Y(E)"=195476.62019501586, "X(N)"=532748.9555589492}, {"Y(E)"=195476.60837096162, "X(N)"=532749.0806443772}, {"Y(E)"=195476.60442441847, "X(N)"=532749.2062254163}, {"Y(E)"=195476.60837096162, "X(N)"=532749.3318064554}, {"Y(E)"=195476.62019501586, "X(N)"=532749.4568918834}, {"Y(E)"=195476.639849917, "X(N)"=532749.5809880454}, {"Y(E)"=195476.66725809622, "X(N)"=532749.7036051906}, {"Y(E)"=195476.7023113859, "X(N)"=532749.824259405}, {"Y(E)"=195476.7448714467, "X(N)"=532749.9424745217}, {"Y(E)"=195476.79477031354, "X(N)"=532750.0577839994}, {"Y(E)"=195476.85181105838, "X(N)"=532750.1697327645}, {"Y(E)"=195476.91576856747, "X(N)"=532750.2778790062}, {"Y(E)"=195476.98639042972, "X(N)"=532750.3817959209}, {"Y(E)"=195477.0633979329, "X(N)"=532750.4810733958}, {"Y(E)"=195477.14648716364, "X(N)"=532750.5753196281}, {"Y(E)"=195477.2353302066, "X(N)"=532750.6641626711}, {"Y(E)"=195477.32957643896, "X(N)"=532750.7472519018}, {"Y(E)"=195477.42885391388, "X(N)"=532750.824259405}, {"Y(E)"=195477.53277082852, "X(N)"=532750.8948812673}, {"Y(E)"=195477.64091707027, "X(N)"=532750.9588387763}, {"Y(E)"=195477.75286583535, "X(N)"=532751.0158795213}, {"Y(E)"=195477.8681753131, "X(N)"=532751.0657783881}, {"Y(E)"=195477.98639042972, "X(N)"=532751.1083384489}, {"Y(E)"=195478.10704464413, "X(N)"=532751.1433917385}, {"Y(E)"=195478.22966178932, "X(N)"=532751.1707999178}, {"Y(E)"=195478.35375795135, "X(N)"=532751.1904548189}, {"Y(E)"=195478.47884337942, "X(N)"=532751.2022788732}, {"Y(E)"=195478.60442441847, "X(N)"=532751.2062254163}]}, {"TM array"=[{"Y(E)"=195478.60442441847, "X(N)"=532752.2062254163}, {"Y(E)"=195478.79279597706, "X(N)"=532752.2003056016}, {"Y(E)"=195478.98042411916, "X(N)"=532752.1825695202}, {"Y(E)"=195479.16656836224, "X(N)"=532752.1530871685}, {"Y(E)"=195479.35049407996, "X(N)"=532752.1119748997}, {"Y(E)"=195479.5314754016, "X(N)"=532752.0593949652}, {"Y(E)"=195479.70879807652, "X(N)"=532751.995554874}, {"Y(E)"=195479.88176229317, "X(N)"=532751.9207065736}, {"Y(E)"=195480.04968544078, "X(N)"=532751.8351454564}, {"Y(E)"=195480.2119048034, "X(N)"=532751.7392091928}, {"Y(E)"=195480.36778017535, "X(N)"=532751.6332763993}, {"Y(E)"=195480.51669638773, "X(N)"=532751.5177651446}, {"Y(E)"=195480.65806573626, "X(N)"=532751.3931312986}, {"Y(E)"=195480.79133030074, "X(N)"=532751.259866734}, {"Y(E)"=195480.9159641468, "X(N)"=532751.1184973855}, {"Y(E)"=195481.0314754016, "X(N)"=532750.9695811732}, {"Y(E)"=195481.13740819498, "X(N)"=532750.8137058013}, {"Y(E)"=195481.2333444586, "X(N)"=532750.6514864386}, {"Y(E)"=195481.31890557587, "X(N)"=532750.483563291}, {"Y(E)"=195481.39375387615, "X(N)"=532750.3105990743}, {"Y(E)"=195481.45759396735, "X(N)"=532750.1332763993}, {"Y(E)"=195481.51017390186, "X(N)"=532749.9522950777}, {"Y(E)"=195481.55128617067, "X(N)"=532749.76836936}, {"Y(E)"=195481.58076852243, "X(N)"=532749.582225117}, {"Y(E)"=195481.59850460375, "X(N)"=532749.3945969748}, {"Y(E)"=195481.60442441847, "X(N)"=532749.2062254163}, {"Y(E)"=195481.59850460375, "X(N)"=532749.0178538577}, {"Y(E)"=195481.58076852243, "X(N)"=532748.8302257155}, {"Y(E)"=195481.55128617067, "X(N)"=532748.6440814725}, {"Y(E)"=195481.51017390186, "X(N)"=532748.4601557548}, {"Y(E)"=195481.45759396735, "X(N)"=532748.2791744332}, {"Y(E)"=195481.39375387615, "X(N)"=532748.1018517582}, {"Y(E)"=195481.31890557587, "X(N)"=532747.9288875415}, {"Y(E)"=195481.2333444586, "X(N)"=532747.760964394}, {"Y(E)"=195481.13740819498, "X(N)"=532747.5987450313}, {"Y(E)"=195481.0314754016, "X(N)"=532747.4428696594}, {"Y(E)"=195480.9159641468, "X(N)"=532747.293953447}, {"Y(E)"=195480.79133030074, "X(N)"=532747.1525840985}, {"Y(E)"=195480.65806573626, "X(N)"=532747.019319534}, {"Y(E)"=195480.51669638773, "X(N)"=532746.894685688}, {"Y(E)"=195480.36778017535, "X(N)"=532746.7791744332}, {"Y(E)"=195480.2119048034, "X(N)"=532746.6732416397}, {"Y(E)"=195480.04968544078, "X(N)"=532746.5773053762}, {"Y(E)"=195479.88176229317, "X(N)"=532746.4917442589}, {"Y(E)"=195479.70879807652, "X(N)"=532746.4168959586}, {"Y(E)"=195479.5314754016, "X(N)"=532746.3530558674}, {"Y(E)"=195479.35049407996, "X(N)"=532746.3004759329}, {"Y(E)"=195479.16656836224, "X(N)"=532746.2593636641}, {"Y(E)"=195478.98042411916, "X(N)"=532746.2298813123}, {"Y(E)"=195478.79279597706, "X(N)"=532746.212145231}, {"Y(E)"=195478.60442441847, "X(N)"=532746.2062254163}, {"Y(E)"=195478.4160528599, "X(N)"=532746.212145231}, {"Y(E)"=195478.2284247178, "X(N)"=532746.2298813123}, {"Y(E)"=195478.0422804747, "X(N)"=532746.2593636641}, {"Y(E)"=195477.858354757, "X(N)"=532746.3004759329}, {"Y(E)"=195477.67737343535, "X(N)"=532746.3530558674}, {"Y(E)"=195477.50005076043, "X(N)"=532746.4168959586}, {"Y(E)"=195477.32708654378, "X(N)"=532746.4917442589}, {"Y(E)"=195477.15916339617, "X(N)"=532746.5773053762}, {"Y(E)"=195476.99694403354, "X(N)"=532746.6732416397}, {"Y(E)"=195476.8410686616, "X(N)"=532746.7791744332}, {"Y(E)"=195476.69215244922, "X(N)"=532746.894685688}, {"Y(E)"=195476.55078310068, "X(N)"=532747.019319534}, {"Y(E)"=195476.4175185362, "X(N)"=532747.1525840985}, {"Y(E)"=195476.29288469013, "X(N)"=532747.293953447}, {"Y(E)"=195476.17737343535, "X(N)"=532747.4428696594}, {"Y(E)"=195476.07144064197, "X(N)"=532747.5987450313}, {"Y(E)"=195475.97550437835, "X(N)"=532747.760964394}, {"Y(E)"=195475.88994326108, "X(N)"=532747.9288875415}, {"Y(E)"=195475.8150949608, "X(N)"=532748.1018517582}, {"Y(E)"=195475.7512548696, "X(N)"=532748.2791744332}, {"Y(E)"=195475.6986749351, "X(N)"=532748.4601557548}, {"Y(E)"=195475.65756266628, "X(N)"=532748.6440814725}, {"Y(E)"=195475.62808031452, "X(N)"=532748.8302257155}, {"Y(E)"=195475.6103442332, "X(N)"=532749.0178538577}, {"Y(E)"=195475.60442441847, "X(N)"=532749.2062254163}, {"Y(E)"=195475.6103442332, "X(N)"=532749.3945969748}, {"Y(E)"=195475.62808031452, "X(N)"=532749.582225117}, {"Y(E)"=195475.65756266628, "X(N)"=532749.76836936}, {"Y(E)"=195475.6986749351, "X(N)"=532749.9522950777}, {"Y(E)"=195475.7512548696, "X(N)"=532750.1332763993}, {"Y(E)"=195475.8150949608, "X(N)"=532750.3105990743}, {"Y(E)"=195475.88994326108, "X(N)"=532750.483563291}, {"Y(E)"=195475.97550437835, "X(N)"=532750.6514864386}, {"Y(E)"=195476.07144064197, "X(N)"=532750.8137058013}, {"Y(E)"=195476.17737343535, "X(N)"=532750.9695811732}, {"Y(E)"=195476.29288469013, "X(N)"=532751.1184973855}, {"Y(E)"=195476.4175185362, "X(N)"=532751.259866734}, {"Y(E)"=195476.55078310068, "X(N)"=532751.3931312986}, {"Y(E)"=195476.69215244922, "X(N)"=532751.5177651446}, {"Y(E)"=195476.8410686616, "X(N)"=532751.6332763993}, {"Y(E)"=195476.99694403354, "X(N)"=532751.7392091928}, {"Y(E)"=195477.15916339617, "X(N)"=532751.8351454564}, {"Y(E)"=195477.32708654378, "X(N)"=532751.9207065736}, {"Y(E)"=195477.50005076043, "X(N)"=532751.995554874}, {"Y(E)"=195477.67737343535, "X(N)"=532752.0593949652}, {"Y(E)"=195477.858354757, "X(N)"=532752.1119748997}, {"Y(E)"=195478.0422804747, "X(N)"=532752.1530871685}, {"Y(E)"=195478.2284247178, "X(N)"=532752.1825695202}, {"Y(E)"=195478.4160528599, "X(N)"=532752.2003056016}, {"Y(E)"=195478.60442441847, "X(N)"=532752.2062254163}]}]
  out "GNSS data info":T4 {"HDOP" scale=0.0..10.0; "PDOP" scale=0.0..10.0; "2D Acc.m" scale=0.0..10.0; "Latitude" format="%.9f"; "Longitude" format="%.9f"; "3D Acc.m" scale=0.0..10.0}
  in  "gnss tm config":T5(tab)
  out "mode status pecent":i16[](array[numeric]) caption="%"
  out "gnss mode cnt":u32[](array[numeric]) caption="count"
  out "Histogram Graph":cluster{i32[], dbl[]}(graph)
  in  "reset statistics":bool
  out "Min circle R":dbl format="%.2g"
  out "Points size":i32
  out "loop count":i32
  in  "tm data reset":bool
  in  "TMarr-size limit":i32=200
  in  "Ref R size":dbl=1.0 format="%.2f"
  in  "Auto\ncenter":bool
  in  "PinDropMrkr":T6(ring)=enum."red_dot" caption="Pin Drop Marker"
  out "xcenter_TM":dbl
  out "ycenter_TM":dbl
  in  "Lat Dbclk":dbl format="%.11f"
  in  "Lon Dbclk":dbl format="%.11f"
  in  "Center \nupdate s":i32=10
  in  "zoom":dbl(slide) scale=3.0..20.0
  out "Sel NMEA":string
  in  "Sel NMEA type":T7(ring)=enum."$GPGGA"
  in  "GNSS Serial cfg":T8={"Port"="COM10", "rate"=115200}
  in  "GNSS Serial delay":u32=20
  out "Raw NMEA":string
  out "Serial bufferN":u32(graph)
  in  "Local Time offset":u32=9
  in  "Send-Serial config":T9={"NMEA out port"="", "baud rate"=9600}
  in  "Data w sel":bool
  in  "Send Serial delay ms":u32=900
  out "log path":string
  out "TM array":cluster{"Y(E)":dbl, "X(N)":dbl}[](array[cluster])
  out "error out":errorcluster
  in  "Log path":path
  in  "clear Ntrip db":bool
  out "Mount point arr":string[](array[string])
  in  "Ntrip accounts DB index":u32(slide) scale=0.0..9.0
  in  "Ntrip accounts DB":T10[](array[typedef])
  in  "Select Mount points":u16(ring) items=["FKP_V31", "SSRG", "VRS_V31", "VRS_V32"]
  out "RTCM recv":string
  out "SourceTable recv-str":string
  in  "update mount point":bool
  out "NMEA cluster":T11
  out "RTCM arr":u8[](array[numeric]) format="%02x"
  out "Version Numbers":T12
  # "Made by ybbaek https://github.com/yunbum"
  # "RL Connect"
  # "under construction"
  # "Network Settings"
  # "Commands"
  # "HW block"
  # "<Common>\n- Log path: C:\\RLmodel_cfg\\Log\n- Config file: C:\\RLmodel_cfg\\Config\n\n<RTK>\n- fkp/vrs mode: Enable GNSS Start before Ntrip Connect\n\n<Google map>\n- Network connection is needed"
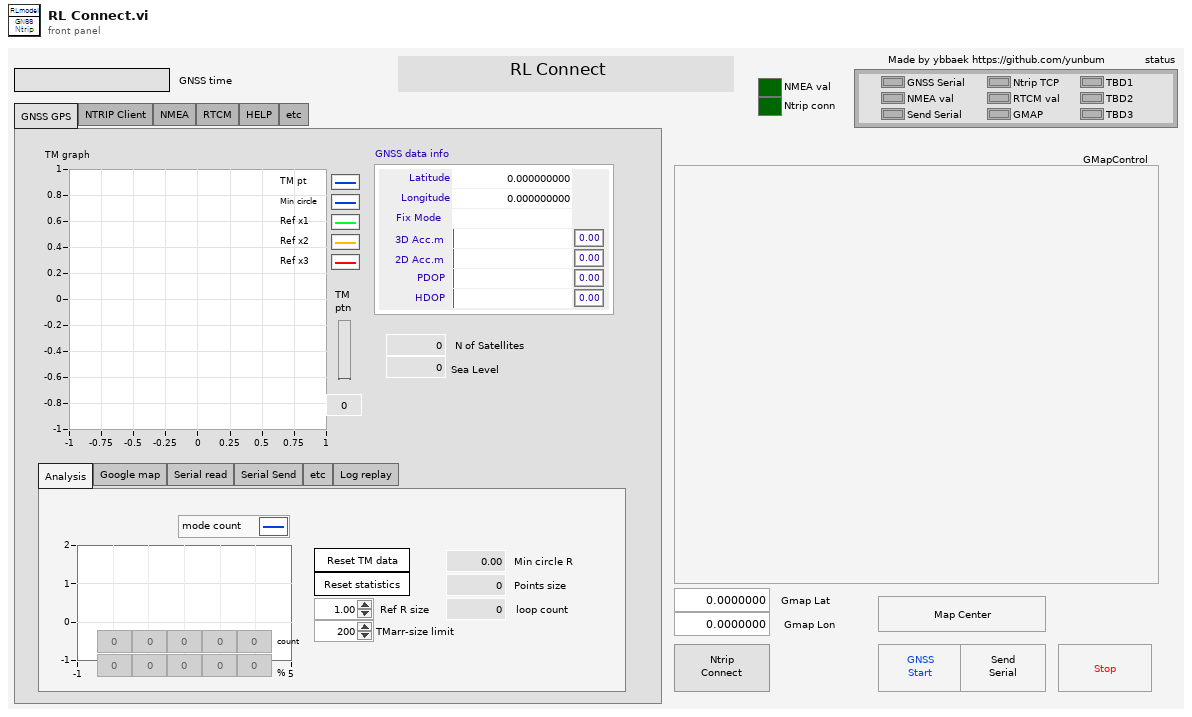
[diagram p1: front panel]
types:
  T1 = typedef "Ntrip error-leds.ctl" = cluster{"GNSS Serial":u8, "NMEA val":u8, "Send Serial":u8, "Ntrip TCP":u8, "RTCM val":u8, "GMAP":u8, "TBD1":u8, "TBD2":u8, "TBD3":u8}
  T2 = enum32{"GNSS GPS", "NTRIP Client", "NMEA", "RTCM", "HELP", "etc"}
  T3 = cluster{"TM array":cluster{"Y(E)":dbl, "X(N)":dbl}[]}[]
  T4 = typedef "ublox-ui_main.ctl" = cluster{"Latitude":dbl, "Longitude":dbl, "Fix Mode":string, "3D Acc.m":dbl, "2D Acc.m":dbl, "PDOP":dbl, "HDOP":dbl}
  T5 = enum32{"Analysis", "Google map", "Serial read", "Serial Send", "etc", "Log replay"}
  T6 = enum16{"none", "arrow", "blue", "blue_small", "blue_dot", "blue_pushpin", "brown_small", "gray_small", "green", "green_small", "green_dot", "green_pushpin", "green_big_go", "yellow", "yellow_small", "yellow_dot", "yellow_big_pause", "yellow_pushpin", "lightblue", "lightblue_dot", "lightblue_pushpin", "orange", "orange_small", "orange_dot", "pink", "pink_dot", "pink_pushpin", "purple", "purple_small", "purple_dot", "purple_pushpin", "red", "red_small", "red_dot", "red_pushpin", "red_big_stop", "black_small", "white_small"}
  T7 = enum16{"$GPGSV", "$GLGSV", "$GPGGA", "$GAGSV", "$GBGSV", "$GNGLL", "$GNGGA", "$GNGSA", "$GNRMC", "$GNVTG"}
  T8 = typedef "gnss_config-2.ctl" = cluster{"Port":refnum<visa-resource-name>, "rate":u32}
  T9 = cluster{"NMEA out port":refnum<visa-resource-name>, "baud rate":u32}
  T10 = typedef "Ntrip_Account_db.ctl" = cluster{"address":string, "port ":u16, "id":string, "pwd":string, "ref pt":string}
  T11 = cluster{"GxGGA":string, "GxGSV":string, "GNRMC":string, "GxTXT":string, "GxGSA":string, "GxGLL":string}
  T12 = cluster{"Major":i32, "Minor":i32, "Patch":i32, "Build":i32}
  T13 = enum16{"Config Save", "Config Load", "LastRUN Save", "LastRUN Load"}
  T14 = typedef "cmd_common.ctl" = enum16{"read", "write"}
  T15 = enum8{"Enabled", "Disabled", "Disabled and Grayed Out"}
  T16 = typedef "cmd_ini-RW.ctl" = enum16{"ini", "read", "write"}
  T17 = typedef "cmd_ini-add-read.ctl" = enum16{"ini", "add", "read"}
  T18 = typedef "GNSS-Ntrip ref.ctl" = cluster{"Mount point arr":refnum<vi>, "Select Mount points":refnum<vi>}
  T19 = typedef "GNSS-Ntrip config.ctl" = cluster{"Ntrip accounts DB":T10[], "Mount points":u16, "Ref r size":dbl, "TMarr limit":i32, "Sel NMEA type":enum16{"$GPGSV", "$GLGSV", "$GPGGA", "$GAGSV", "$GBGSV", "$GNGLL", "$GNGGA", "$GNGSA", "$GNRMC", "$GNVTG"}, "Local Time offset":u32, "GNSS Serial delay":u32, "Send Serial delay":u32, "Send Serial config":cluster{"NMEA out port":refnum<visa-resource-name>, "baud rate":u32}, "Mount point arr":string[], "Ntrip account DB index":u32}
  T20 = cluster{"NA":u32, "valid":u32, "DGPS":u32, "RTK float":u32, "RTK fixed":u32}
  T21 = cluster{"Gmap Lat":refnum<vi>, "Gmap Lon":refnum<vi>, "Lat Dbclk":refnum<vi>, "Lon Dbclk":refnum<vi>, "zoom":refnum<vi>, "PinDropMrkr":refnum<vi>}
  T22 = typedef "GNSS-Ntrip process val.ctl" = cluster{"GNSS time":string, "Ntrip conn":bool, "NMEA val":bool, "ycenter_TM":dbl, "xcenter_TM":dbl, "TM ref circles":cluster{"Y(E)":dbl, "X(N)":dbl}[], "RTCM recv-str":string, "GNSS Serail buff N":u32, "Sel NMEA type":enum16{"$GPGSV", "$GLGSV", "$GPGGA", "$GAGSV", "$GBGSV", "$GNGLL", "$GNGGA", "$GNGSA", "$GNRMC", "$GNVTG"}, "RTCM recv_sourcetable":string, "NMEA cluster":cluster{"GxGGA":string, "GxGSV":string, "GNRMC":string, "GxTXT":string, "GxGSA":string, "GxGLL":string}, "Sel NMEA str":string, "NMEA recv-str":string}
  T23 = typedef "gmap_fgv-cmd.ctl" = enum16{"marker type change", "save_image", "coll of points", "zoom n center markers", "add overlay reference", "read", "zoom", "set position by keyword", "set map provider", "map provider update", "create", "add marker", "clear marker", "close"}
  T24 = typedef "error_state-val.ctl" = enum16{"na", "error", "OK"}
  T25 = typedef "NMEA.lvlib/NMEA_LatitudeDirection.ctl" = enum16{"", "North", "South"}
  T26 = typedef "NMEA.lvlib/NMEA_LongitudeDirection.ctl" = enum16{"", "East", "West"}
  T27 = typedef "NMEA.lvlib/NMEA_GPS-Quality.ctl" = enum16{"Invalid", "GPS fix (SPS)", "DGPS fix", "PPS fix", "Real Time Kinematic", "Float RTK", "estimated", "Manual input mode", "Simulation mode"}
  T28 = cluster{"$GPGGA-message_OUT":cluster{"TimeStamp":timestamp, "Latitude":dbl, "Latitude-Direction":T25, "Longitude":dbl, "Longitude-Direction":T26, "GPS-Quality":T27, "N of Satellites":i32, "HDOP":dbl, "Altitude above Mean-Sea-Level":dbl, "Geoidal separation":dbl, "Time since last DGPS update":dbl, "DGPS reference station ID":i32}}
  T29 = cluster{"TM array":cluster{"Y(E)":dbl, "X(N)":dbl}[]}
  T30 = cluster{"Ntrip tcp":bool, "GNSS serial":bool, "RTCM serial":bool, "Send serial":bool}
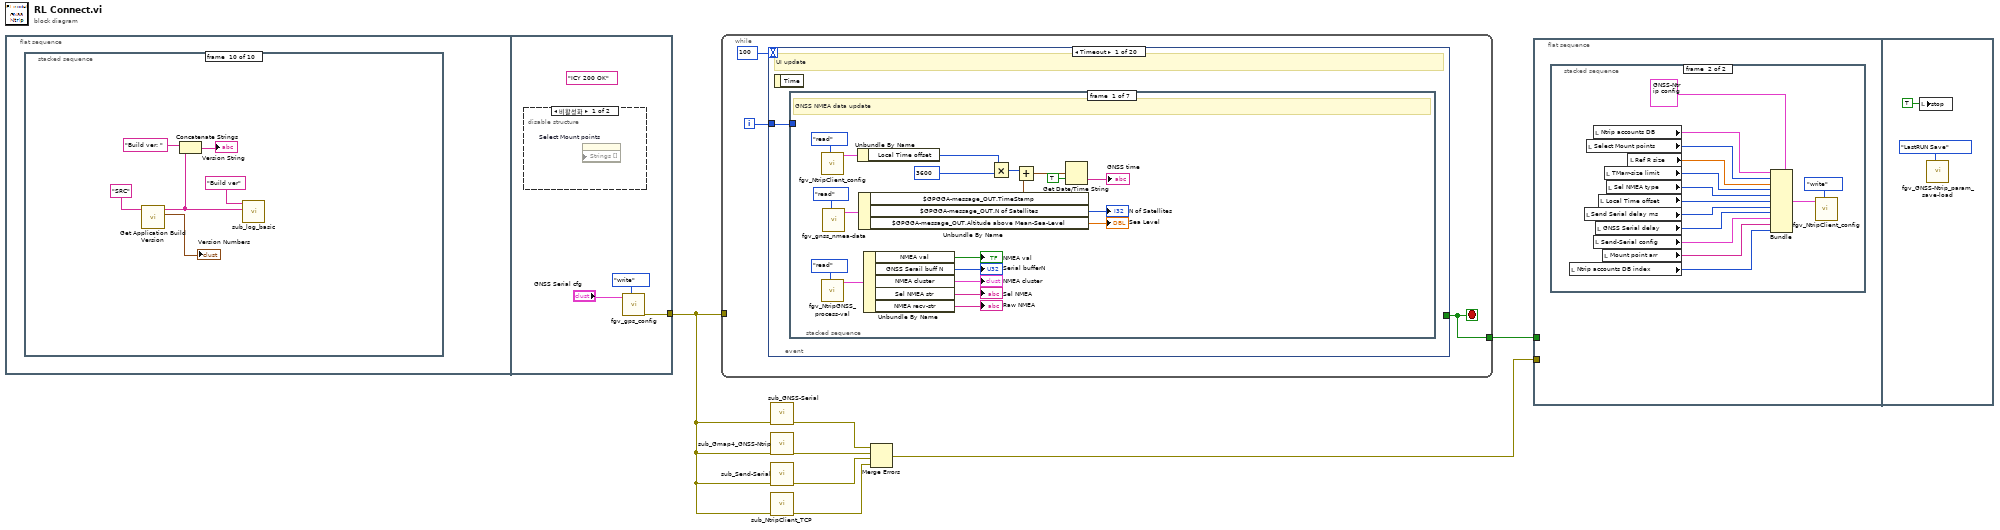
[diagram p0: block diagram]
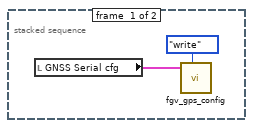
[diagram p2: hidden frame]
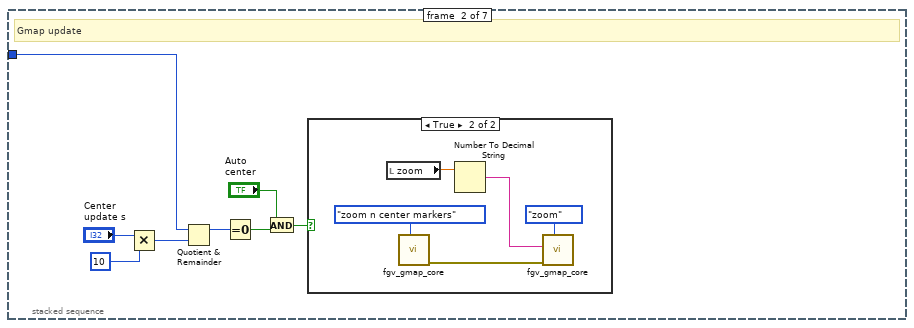
[diagram p3: hidden frame]
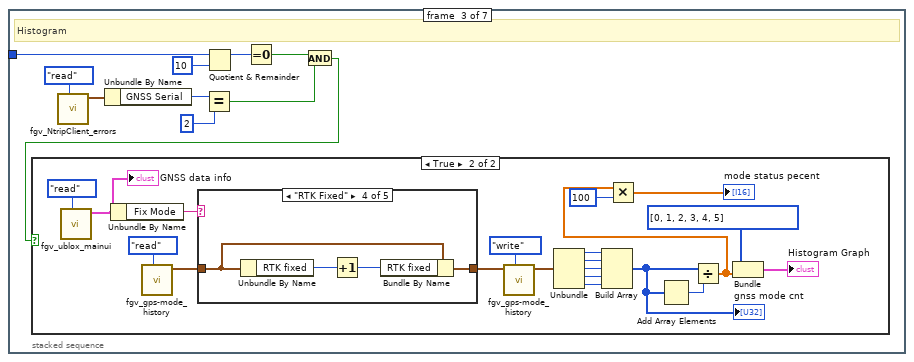
[diagram p5: hidden frame]
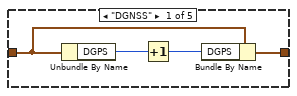
[diagram p7: hidden frame]
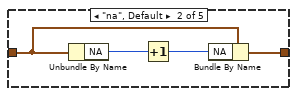
[diagram p8: hidden frame]
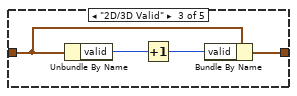
[diagram p9: hidden frame]
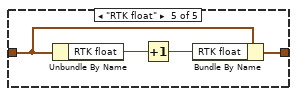
[diagram p10: hidden frame]
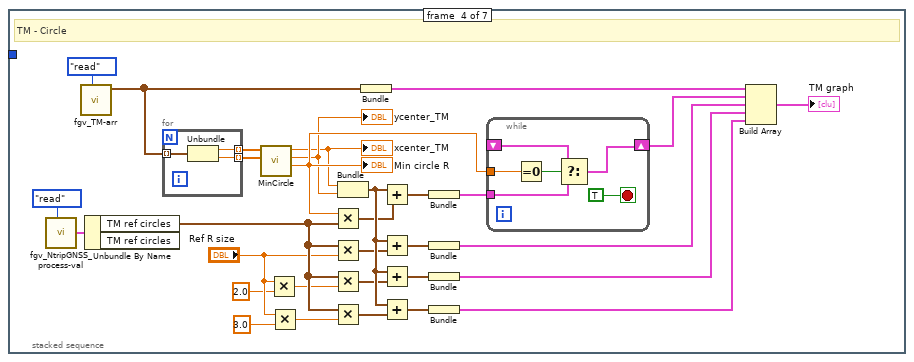
[diagram p11: hidden frame]
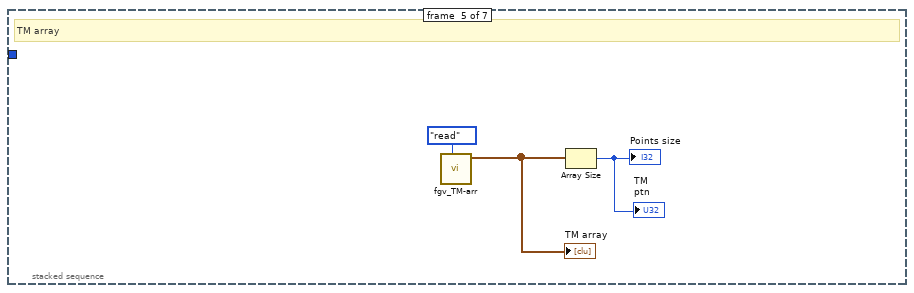
[diagram p12: hidden frame]
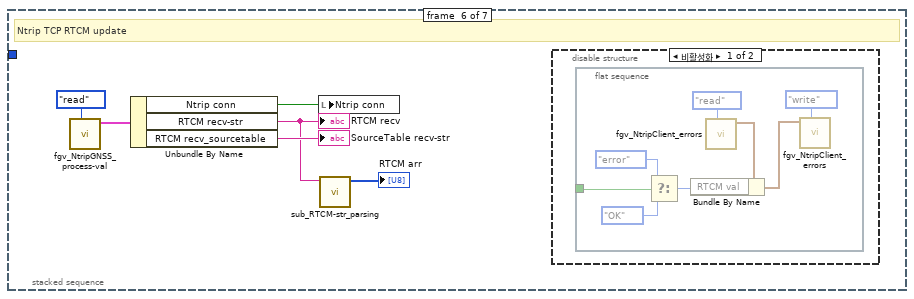
[diagram p13: hidden frame]
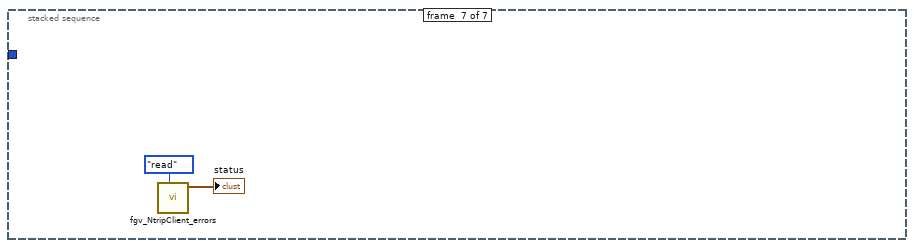
[diagram p15: hidden frame]
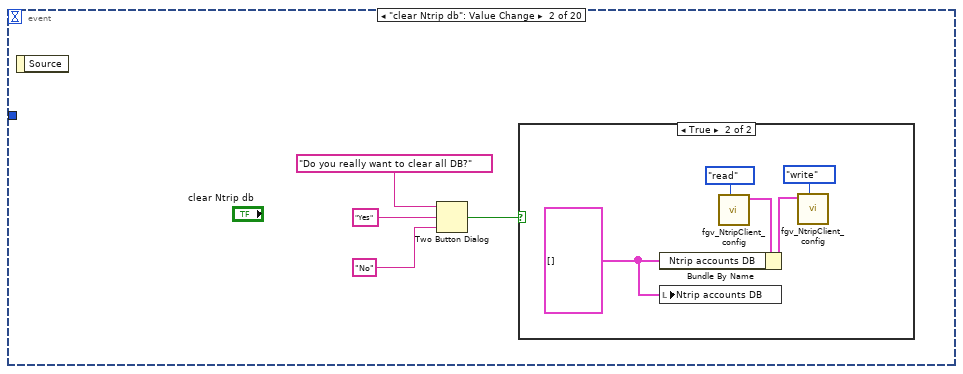
[diagram p16: hidden frame]
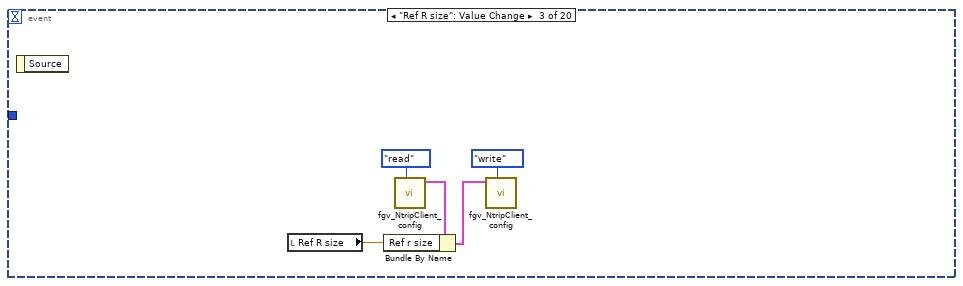
[diagram p18: hidden frame]
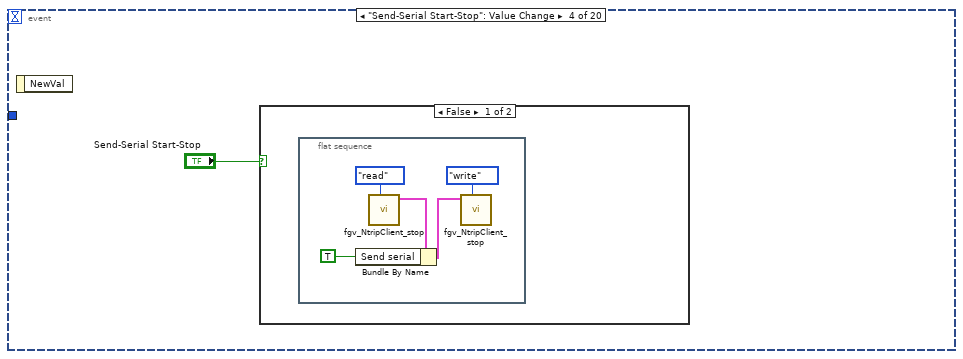
[diagram p19: hidden frame]
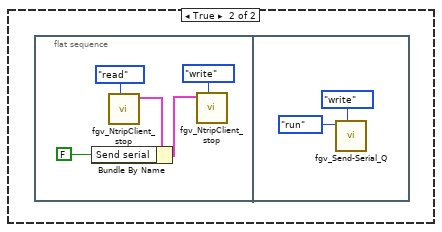
[diagram p20: hidden frame]
diagram:
  n1 = flat-sequence {
    tunnel: [w97] -> w6
    frame #0 {
      n2 = stacked-sequence {
        frame #0 {
          n3 = call "fgv_GNSS-Ntrip_param_save-load.vi"("ctl"=T13."LastRUN Load") -> ("error out"=w8:errorcluster)  [unwired: 9 in, 1 out]
          n4 = stacked-sequence {
            tunnel: w8 -> [_ _ _]
            frame #0 {
              n5 = call "fgv_gps_config.vi"("cmd"=enum16{"read", "write"}."read") -> ("GNSS cfg out"=w10:T8)  [unwired: 9 in, 1 out]
              n6 = local write "GNSS Serial cfg"(w10) -> ()
            }
            frame #1 {
              n7 = call "fgv_NtripClient_config.vi"("cmd"=cmd_common."read") -> ("config val out"=w24:T19)  [unwired: 10 in]
              n8 = Unbundle(w24) -> ("Ntrip accounts DB"=w22:T10[], "Mount points"=w21:u16, "Ref r size"=w20:dbl, "TMarr limit"=w19:i32, "Sel NMEA type"=w16:T7, "Local Time offset"=w15:u32, "GNSS Serial delay"=w14:u32, "Send Serial delay"=w23:u32, "Send Serial config"=w17:T9, "Mount point arr"=w18:string[], "Ntrip account DB index"=w12:u32)
              n9 = Build Array(w12) -> (w13:u32[])
              n10 = local write "Select Mount points"(w12) -> ()
              n11 = property on="Ntrip accounts DB" class="Arr (strict)"("Index Values"=w13) -> ()  [unwired: 2 in, 2 out]
              n12 = local write "Ntrip accounts DB index"(w12) -> ()
              n13 = local write "Send Serial delay ms"(w23) -> ()
              n14 = local write "Select Mount points"(w21) -> ()
              n15 = local write "Ntrip accounts DB"(w22) -> ()
              n16 = local write "Send-Serial config"(w17) -> ()
              n17 = local write "GNSS Serial delay"(w14) -> ()
              n18 = local write "Local Time offset"(w15) -> ()
              n19 = local write "Mount point arr"(w18) -> ()
              n20 = local write "TMarr-size limit"(w19) -> ()
              n21 = property on="Select Mount points" class="Ring (strict)"("Strings []"=w18) -> ()  [unwired: 2 in, 2 out]
              n22 = local write "Sel NMEA type"(w16) -> ()
              n23 = local write "Ref R size"(w20) -> ()
            }
            frame #2 {
              n24 = property on="Select Mount points" class="Ring (strict)"("DisabledEnum"=T15."Disabled and Grayed Out" ("비활성화")) -> ()  [unwired: 2 in, 2 out]
            }
          }
        }
        frame #1 {
          n25 = call "fgv_global-stop.vi"("cmd"=enum16{"init", "stop", "read"}."init") -> ()  [unwired: 10 in, 1 out]
          n26 = call "fgv_gps-mode_history.vi"("cmd"=cmd_ini-RW."ini") -> ("data out"=w27:T20)  [unwired: 10 in]
          n27 = call "fgv_RTCM_TCP_Q.vi"("cmd"=enum16{"create", "write", "read", "close"}."create") -> ()  [unwired: 9 in, 2 out]
          n28 = Unbundle(w27) -> ("NA"=w29:u32, "valid"=w33:u32, "DGPS"=w32:u32, "RTK float"=w31:u32, "RTK fixed"=w30:u32)
          n29 = call "fgv_TM-arr.vi"("cmd"=cmd_ini-add-read."ini") -> ()  [unwired: 10 in, 1 out]
          n30 = call "fgv_Send-Serial_Q.vi"("cmd"=enum16{"create", "write", "read", "close"}."create") -> ()  [unwired: 9 in, 2 out]
          n31 = Build Array(w29, w33, w32, w31, w30) -> (w28:u32[])
          n32 = call "fgv_NtripGNSS_process-val.vi"("cmd"=cmd_ini-RW."ini") -> ()  [unwired: 10 in, 1 out]
          n33 = call "fgv_GNSS_Serial_Q.vi"("cmd"=enum16{"create", "write", "read", "close"}."create") -> ()  [unwired: 9 in, 2 out]
          n34 = local write "gnss mode cnt"(w28) -> ()
          n35 = call "fgv_NtripClient_stop.vi"("cmd"=cmd_ini-RW."ini") -> ()  [unwired: 10 in, 1 out]
          n36 = call "fgv_NtripClient_errors.vi"("cmd"=enum16{"init", "read", "write"}."init") -> ()  [unwired: 9 in, 2 out]
        }
        frame #2 {
          n37 = control-ref of="Gmap Lat"() -> (w50:refnum<vi>)
          n38 = control-ref of="Gmap Lon"() -> (w51:refnum<vi>)
          n39 = control-ref of="Lat Dbclk"() -> (w52:refnum<vi>)
          n40 = control-ref of="Lon Dbclk"() -> (w53:refnum<vi>)
          n41 = control-ref of="PinDropMrkr"() -> (w55:refnum<vi>)
          n42 = control-ref of="zoom"() -> (w54:refnum<vi>)
          n43 = control-ref of="Mount point arr"() -> (w47:refnum<vi>)
          n44 = control-ref of="Select Mount points"() -> (w44:refnum<vi>)
          n45 = Bundle("Gmap Lat"=w50, "Gmap Lon"=w51, "Lat Dbclk"=w52, "Lon Dbclk"=w53, "zoom"=w54, "PinDropMrkr"=w55) -> (w56:T21)  [unwired: 1 in]
          n46 = Bundle(cluster=T18 {"Mount point arr"=refnum, "Select Mount points"=refnum} ("ref 2"), "Mount point arr"=w47, "Select Mount points"=w44) -> (w45:T18)
          n47 = call "fgv_ctr-ref_gmap.vi"("cmd"=cmd_common."write", "ref in"=w56) -> ()  [unwired: 9 in, 1 out]
          n48 = call "fgv_ctrl-ref_cluster.vi"("cmd"=enum16{"read", "write"}."write", "ref"=w56) -> ()  [unwired: 9 in, 1 out]
          n49 = call "fgv_GNSS-Ntrip_ctrl-refs.vi"("cmd"=cmd_common."write", "ref"=w45) -> ()  [unwired: 9 in, 1 out]
        }
        frame #3 {
          n50 = call "fgv_NtripClient_config.vi"("cmd"=cmd_common."read") -> ("config val out"=w61:T19)  [unwired: 10 in]
          n51 = Bundle By Name(cluster=w61, "Send Serial config"="Send-Serial config") -> (w60:T19)
          n52 = call "fgv_NtripClient_config.vi"("cmd"=cmd_common."write", "config val"=w60) -> ()  [unwired: 9 in, 1 out]
        }
        frame #4 {
          n53 = call "sub_gmap_init.vi"("GMapControl"="GMapControl") -> ()  [unwired: 10 in, 1 out]
        }
        frame #5 {
          n54 = call "sub_log_fine-name.vi"("Sel"=enum16{"SRC", "RL Connect"}."RL Connect") -> ("log path"=w63:string)  [unwired: 10 in]
          "log path" <- w63
          n55 = call "sub_log_basic.vi"("desc"=w63, "Title"="log ptah") -> ()  [unwired: 9 in, 1 out]
        }
        frame #6 {
          w67 = 100
          n56 = Increment(x=w67) -> (x+1=w74:i32)
          n57 = Divide(x=6.283185307179586, y=w67) -> (x/y=w73:dbl)
          n58 = for {
            N: w74 -> [_]
            tunnel: w73 -> [w79]
            tunnel: [w75] -> w70 mode=indexing
            i -> [w80]
            n59 = Multiply(x=w79, y=w80) -> (x*y=w78:dbl)
            n60 = Sine & Cosine(0:w78) -> (1:w77:dbl, 2:w76:dbl)
            n61 = Bundle(w77, w76) -> (w75:cluster{dbl, dbl})  [unwired: 1 in]
          }
          n62 = call "fgv_NtripGNSS_process-val.vi"("cmd"=cmd_ini-RW."read") -> ("process val out"=w72:T22)  [unwired: 10 in]
          n63 = Bundle By Name(cluster=w72, "TM ref circles"=w70) -> (w71:T22)
          n64 = call "fgv_NtripGNSS_process-val.vi"("cmd"=cmd_ini-RW."write", "process val"=w71) -> ()  [unwired: 9 in, 1 out]
        }
        frame #7 {
          w82 = "" ("read raw")
          w84 = FALSE ("정지")
          n65 = disable-structure shown="비활성화" {
            frame Disabled {
              n66 = local write "Ntrip accounts DB index"(u32 0 ("Ntrip accounts DB index")) -> ()
            }
            frame Enabled {
            }
          }
          n67 = local write "Histogram Graph"(cluster{i32[], dbl[]} {[], []} ("Histogram Graph")) -> ()
          n68 = local write "Raw NMEA"(w82) -> ()
          n69 = local write "Sel NMEA"(w82) -> ()
          n70 = local write "RTCM recv"(w82) -> ()
          n71 = local write "SourceTable recv-str"(w82) -> ()
          n72 = local write "stop"(w84) -> ()
          n73 = local write "GNSS Start-Stop"(w84) -> ()
          n74 = local write "Send-Serial Start-Stop"(w84) -> ()
          n75 = local write "Ntrip connect"(w84) -> ()
          "Ntrip conn" <- FALSE ("ntrip val")
          "error out" <- errorcluster {"status"=FALSE, "code"=0, "source"=""} ("error out")
        }
        frame #8 {
          w87 = T15."Enabled" ("Disabled")
          n76 = property on="TM\nptn" class="Slide (strict)"("Scale.Marker.Selection End"="TMarr-size limit") -> ()  [unwired: 2 in, 2 out]
          n77 = property on="Select Mount points" class="Ring (strict)"("DisabledEnum"=T15."Disabled and Grayed Out" ("비활성화")) -> ()  [unwired: 2 in, 2 out]
          n78 = property on="Ntrip accounts DB index" class="Slide (strict)"("DisabledEnum"=w87) -> ()  [unwired: 2 in, 2 out]
          n79 = property on="Ntrip accounts DB" class="Arr (strict)"("DisabledEnum"=w87) -> ()  [unwired: 2 in, 2 out]
          n80 = property on="update mount point" class="Bool"("DisabledEnum"=w87) -> ()  [unwired: 2 in, 2 out]
        }
        frame #9 {
          n81 = call "Get Application Build Version.vi"("Project Filename"="SRC") -> ("Version Numbers"=→"Version Numbers":T12, "Version String"=w90:string)  [unwired: 8 in, 1 out]
          n82 = Concatenate Strings("Build ver: " ("string"), w90) -> (→"Version String":string)
          n83 = call "sub_log_basic.vi"("desc"=w90, "Title"="Build ver") -> ()  [unwired: 9 in, 1 out]
        }
      }
    }
    frame #1 {
      (unwired) "ICY 200 OK" ("정규식")
      n84 = disable-structure shown="비활성화" {
        frame Disabled {
          n85 = property on="Select Mount points" class="Ring (strict)" props=["Strings []"]() -> ()  [unwired: 3 in, 2 out]
        }
        frame Enabled {
        }
      }
      n86 = call "fgv_gps_config.vi"("cmd"=enum16{"read", "write"}."write", "GNSS cfg"="GNSS Serial cfg") -> ("error out"=w97:errorcluster)  [unwired: 8 in, 1 out]
    }
  }
  n87 = while {
    tunnel: w6 -> [_]
    tunnel: [w101] -> w7
    i -> [w99]
    stop <- w101 stop-if-true
    n88 = event shown="[0] Timeout" {
      selector: _ -> [_ _ _ _ _ _ _ _ _ _ _ _ _ _ _ _ _ _ _ _]
      dyn-events: _ -> [_ _ _ _ _ _ _ _ _ _ _ _ _ _ _ _ _ _ _ _]
      timeout: 100 -> [_ _ _ _ _ _ _ _ _ _ _ _ _ _ _ _ _ _ _ _]
      tunnel: [_ _ _ _ _ _ _ _ _ _ _ w330 _ _ _ _ _ _ _ _] -> w101
      tunnel: w99 -> [w102 _ _ _ _ _ _ _ _ _ _ _ _ _ _ _ _ _ _ _]
      event Timeout {
        # "UI update"
        n89 = event-data() -> ()  [unwired: 1 in, 1 out]
        n90 = stacked-sequence {
          tunnel: w102 -> [_ w123 w144 _ _ _ _]
          frame #0 {
            # "GNSS NMEA data update"
            n91 = call "fgv_NtripClient_config.vi"("cmd"=cmd_common."read") -> ("config val out"=w115:T19)  [unwired: 10 in]
            n92 = call "fgv_NtripGNSS_process-val.vi"("cmd"=cmd_ini-RW."read") -> ("process val out"=w106:T22)  [unwired: 10 in]
            n93 = call "fgv_gnss_nmea-data.vi"("cmd"=cmd_common."read") -> ("nmea-data out"=w120:T28)  [unwired: 10 in]
            n94 = Unbundle By Name(w115) -> ("Local Time offset"=w114:u32)
            n95 = Unbundle By Name(w120) -> ("$GPGGA-message_OUT.TimeStamp"=w119:timestamp, "$GPGGA-message_OUT.N of Satellites"=→"N of Satellites":i32, "$GPGGA-message_OUT.Altitude above Mean-Sea-Level"=→"Sea Level":dbl)
            n96 = Unbundle By Name(w106) -> ("NMEA val"=→"NMEA val":bool, "GNSS Serail buff N"=→"Serial bufferN":u32, "NMEA cluster"=→"NMEA cluster":T11, "Sel NMEA str"=→"Sel NMEA":string, "NMEA recv-str"=→"Raw NMEA":string)
            n97 = Multiply(x=w114, y=u32 3600) -> (x*y=w122:u32)
            n98 = Add(x=w122, y=w119) -> (x+y=w121:timestamp)
            n99 = Get Date/Time String(seconds (now)=w121, want seconds? (F)=TRUE ("초 보이기? (거짓)")) -> (time string=→"GNSS time":string)  [unwired: 1 in, 1 out]
          }
          frame #1 {
            # "Gmap update"
            n100 = Multiply(x="Center \nupdate s", y=10) -> (x*y=w124:i32)
            n101 = Quotient & Remainder(x=w123, y=w124) -> (x-y*floor(x/y)=w128:i32)  [unwired: 1 out]
            n102 = Equal To 0?(x=w128) -> (x = 0?=w129:bool)
            n103 = And(x="Auto\ncenter", y=w129) -> (x .and. y?=w130:bool)
            n104 = case shown="True" w130 {
              frame False {
              }
              frame True {
                n105 = local read "zoom"() -> (w135:dbl)
                n106 = call "fgv_gmap_core.vi"("cmd"=gmap_fgv-cmd."zoom n center markers") -> ("error out"=w131:errorcluster)  [unwired: 7 in, 3 out]
                n107 = Number To Decimal String(number=w135) -> (decimal integer string=w134:string)  [unwired: 1 in]
                n108 = call "fgv_gmap_core.vi"(7:"cmd"=gmap_fgv-cmd."zoom" ("cmd"), "error in"=w131, 10:"cmd"=w134) -> ()  [unwired: 5 in, 4 out]
              }
            }
          }
          frame #2 {
            # "Histogram"
            n109 = call "fgv_NtripClient_errors.vi"("cmd"=enum16{"init", "read", "write"}."read") -> ("Error led out"=w140:T1)  [unwired: 9 in, 1 out]
            n110 = Unbundle By Name(w140) -> ("GNSS Serial"=w139:u8)
            n111 = Equal?(x=w139, y=u8 2) -> (x = y?=w137:bool)
            n112 = Quotient & Remainder(x=w144, y=10) -> (x-y*floor(x/y)=w145:i32)  [unwired: 1 out]
            n113 = Equal To 0?(x=w145) -> (x = 0?=w142:bool)
            n114 = And(x=w142, y=w137) -> (x .and. y?=w136:bool)
            n115 = case shown="True" w136 {
              frame False {
              }
              frame True {
                n116 = call "fgv_ublox_mainui.vi"("cmd"=cmd_common."read") -> ("MainUI gnss out"=w153:T4)  [unwired: 10 in]
                "GNSS data info" <- w153
                n117 = Unbundle By Name(w153) -> ("Fix Mode"=w154:string)
                n118 = call "fgv_gps-mode_history.vi"("cmd"=cmd_ini-RW."read") -> ("data out"=w155:T20)  [unwired: 10 in]
                n119 = case shown="\"RTK Fixed\"" w154 {
                  tunnel: w155 -> [w169 w173 w177 w181 w185]
                  tunnel: [w168 w172 w176 w180 w184] -> w156
                  frame "DGNSS" {
                    n120 = Unbundle By Name(w169) -> ("DGPS"=w167:u32)
                    n121 = Increment(x=w167) -> (x+1=w166:u32)
                    n122 = Bundle By Name(cluster=w169, "DGPS"=w166) -> (w168:T20)
                  }
                  frame "na", Default {
                    n123 = Unbundle By Name(w173) -> ("NA"=w171:u32)
                    n124 = Increment(x=w171) -> (x+1=w170:u32)
                    n125 = Bundle By Name(cluster=w173, "NA"=w170) -> (w172:T20)
                  }
                  frame "2D/3D Valid" {
                    n126 = Unbundle By Name(w177) -> ("valid"=w175:u32)
                    n127 = Increment(x=w175) -> (x+1=w174:u32)
                    n128 = Bundle By Name(cluster=w177, "valid"=w174) -> (w176:T20)
                  }
                  frame "RTK Fixed" {
                    n129 = Unbundle By Name(w181) -> ("RTK fixed"=w179:u32)
                    n130 = Increment(x=w179) -> (x+1=w178:u32)
                    n131 = Bundle By Name(cluster=w181, "RTK fixed"=w178) -> (w180:T20)
                  }
                  frame "RTK float" {
                    n132 = Unbundle By Name(w185) -> ("RTK float"=w183:u32)
                    n133 = Increment(x=w183) -> (x+1=w182:u32)
                    n134 = Bundle By Name(cluster=w185, "RTK float"=w182) -> (w184:T20)
                  }
                }
                n135 = call "fgv_gps-mode_history.vi"("cmd"=cmd_ini-RW."write", "data"=w156) -> ("data out"=w157:T20)  [unwired: 9 in]
                n136 = Unbundle(w157) -> ("NA"=w158:u32, "valid"=w162:u32, "DGPS"=w161:u32, "RTK float"=w160:u32, "RTK fixed"=w159:u32)
                n137 = Build Array(w158, w162, w161, w160, w159) -> (w165:u32[])
                "gnss mode cnt" <- w165
                n138 = Add Array Elements(numeric array=w165) -> (sum=w164:u32)
                n139 = Divide(x=w165, y=w164) -> (x/y=w147:dbl[])
                n140 = Multiply(x=w147, y=i16 100) -> (x*y=→"mode status pecent":dbl[])
                n141 = Bundle(i32[] [0, 1, 2, 3, 4, 5], w147) -> (→"Histogram Graph":cluster{i32[], dbl[]})  [unwired: 1 in]
              }
            }
          }
          frame #3 {
            # "TM - Circle"
            n142 = call "fgv_NtripGNSS_process-val.vi"("cmd"=cmd_ini-RW."read") -> ("process val out"=w214:T22)  [unwired: 10 in]
            n143 = call "fgv_TM-arr.vi"("cmd"=cmd_ini-add-read."read") -> ("TM array"=w216:cluster{"Y(E)":dbl, "X(N)":dbl}[])  [unwired: 10 in]
            n144 = Unbundle By Name(w214) -> ("TM ref circles"=w215:cluster{"Y(E)":dbl, "X(N)":dbl}[])  [unwired: 1 out]
            n145 = for {
              tunnel: [w225] -> w191 mode=indexing
              tunnel: [w224] -> w192 mode=indexing
              tunnel: w216 -> [w223] mode=indexing
              n146 = Unbundle(w223) -> ("Y(E)"=w225:dbl, "X(N)"=w224:dbl)
            }
            n147 = call "MinCircle.vi"("y"=w192, "x"=w191) -> ("r"=w201:dbl, "yc"=w194:dbl, "xc"=w193:dbl)  [unwired: 6 in, 1 out]
            "xcenter_TM" <- w193
            "ycenter_TM" <- w194
            "Min circle R" <- w201
            n148 = Multiply(x="Ref R size", y=2.0) -> (x*y=w206:dbl)
            n149 = Multiply(x="Ref R size", y=3.0) -> (x*y=w187:dbl)
            n150 = Multiply(x=w201, y=w215) -> (x*y=w195:cluster{"Y(E)":dbl, "X(N)":dbl}[])
            n151 = Multiply(x=w215, y="Ref R size") -> (x*y=w205:cluster{"Y(E)":dbl, "X(N)":dbl}[])
            n152 = Multiply(x=w215, y=w206) -> (x*y=w204:cluster{"Y(E)":dbl, "X(N)":dbl}[])
            n153 = Multiply(x=w215, y=w187) -> (x*y=w207:cluster{"Y(E)":dbl, "X(N)":dbl}[])
            n154 = Bundle("xc"=w193, "yc"=w194) -> (w208:cluster{"xc":dbl, "yc":dbl})  [unwired: 1 in]
            n155 = Bundle("TM array"=w216) -> (w197:T29)  [unwired: 1 in]
            n156 = Add(x=w208, y=w195) -> (x+y=w196:cluster{dbl, dbl}[])
            n157 = Add(x=w208, y=w205) -> (x+y=w202:cluster{dbl, dbl}[])
            n158 = Add(x=w208, y=w204) -> (x+y=w210:cluster{dbl, dbl}[])
            n159 = Add(x=w208, y=w207) -> (x+y=w209:cluster{dbl, dbl}[])
            n160 = Bundle(w196) -> (w199:cluster{cluster{dbl, dbl}[]})  [unwired: 1 in]
            n161 = Bundle(w202) -> (w203:cluster{cluster{dbl, dbl}[]})  [unwired: 1 in]
            n162 = Bundle(w210) -> (w211:cluster{cluster{dbl, dbl}[]})  [unwired: 1 in]
            n163 = Bundle(w209) -> (w212:cluster{cluster{dbl, dbl}[]})  [unwired: 1 in]
            n164 = while {
              shift-right: [w217] -> w200
              shift-left: _ -> [w219]
              tunnel: w201 -> [w221]
              tunnel: w199 -> [w218]
              stop <- TRUE stop-if-true
              n165 = Equal To 0?(x=w221) -> (x = 0?=w220:bool)
              n166 = Select(t=w219, s=w220, f=w218) -> (s? t:f=w217:cluster{cluster{dbl, dbl}[]})
            }
            n167 = Build Array(w197, w200, w203, w211, w212) -> (→"TM graph":T3)
          }
          frame #4 {
            # "TM array"
            n168 = call "fgv_TM-arr.vi"("cmd"=cmd_ini-add-read."read") -> ("TM array"=w226:cluster{"Y(E)":dbl, "X(N)":dbl}[])  [unwired: 10 in]
            "TM array" <- w226
            n169 = Array Size(array=w226) -> (size(s)=→"Points size" →"TM\nptn":i32)
          }
          frame #5 {
            # "Ntrip TCP RTCM update"
            n170 = call "fgv_NtripGNSS_process-val.vi"("cmd"=cmd_ini-RW."read") -> ("process val out"=w231:T22)  [unwired: 10 in]
            n171 = Unbundle By Name(w231) -> ("Ntrip conn"=w232:bool, "RTCM recv-str"=w230:string, "RTCM recv_sourcetable"=→"SourceTable recv-str":string)
            "RTCM recv" <- w230
            n172 = local write "Ntrip conn"(w232) -> ()
            n173 = call "sub_RTCM-str_parsing.vi"("RTCM recv-str"=w230) -> ("RTCM arr"=→"RTCM arr":u8[])  [unwired: 9 in, 1 out]
            n174 = disable-structure shown="비활성화" {
              frame Disabled {
                n175 = flat-sequence {
                  tunnel: _ -> [w238]
                  frame #0 {
                    n176 = Select(t=error_state-val."error", s=w238, f=error_state-val."OK") -> (s? t:f=w235:T24)
                    n177 = call "fgv_NtripClient_errors.vi"("cmd"=enum16{"init", "read", "write"}."read") -> ("Error led out"=w240:T1)  [unwired: 9 in, 1 out]
                    n178 = Bundle By Name(cluster=w240, "RTCM val"=w235) -> (w239:T1)
                    n179 = call "fgv_NtripClient_errors.vi"("cmd"=enum16{"init", "read", "write"}."write", "Error led"=w239) -> ()  [unwired: 8 in, 2 out]
                  }
                }
              }
              frame Enabled {
              }
            }
          }
          frame #6 {
            n180 = call "fgv_NtripClient_errors.vi"("cmd"=enum16{"init", "read", "write"}."read") -> ("Error led out"=→"status":T1)  [unwired: 9 in, 1 out]
          }
        }
      }
      event "clear Ntrip db": Value Change {
        n181 = event-data() -> ()  [unwired: 1 in, 1 out]
        n182 = Two Button Dialog(message="Do you really want to clear all DB?" ("메시지"), 1:"No" ("참 버튼 이름(\"확인\")"), 2:"Yes" ("참 버튼 이름(\"확인\")")) -> (T button?=w245:bool)
        n183 = case shown="True" w245 {
          frame False {
          }
          frame True {
            w249 = T10[] [] ("Ntrip accounts DB")
            n184 = local write "Ntrip accounts DB"(w249) -> ()
            n185 = call "fgv_NtripClient_config.vi"("cmd"=cmd_common."read") -> ("config val out"=w253:T19)  [unwired: 10 in]
            n186 = Bundle By Name(cluster=w253, "Ntrip accounts DB"=w249) -> (w252:T19)
            n187 = call "fgv_NtripClient_config.vi"("cmd"=cmd_common."write", "config val"=w252) -> ()  [unwired: 9 in, 1 out]
          }
        }
      }
      event "Ref R size": Value Change {
        n188 = event-data() -> ()  [unwired: 1 in, 1 out]
        n189 = local read "Ref R size"() -> (w254:dbl)
        n190 = call "fgv_NtripClient_config.vi"("cmd"=cmd_common."read") -> ("config val out"=w258:T19)  [unwired: 10 in]
        n191 = Bundle By Name(cluster=w258, "Ref r size"=w254) -> (w257:T19)
        n192 = call "fgv_NtripClient_config.vi"("cmd"=cmd_common."write", "config val"=w257) -> ()  [unwired: 9 in, 1 out]
      }
      event "Send-Serial Start-Stop": Value Change {
        n193 = event-data() -> ()  [unwired: 1 in, 1 out]
        n194 = case shown="False" "Send-Serial Start-Stop" {
          frame False {
            n195 = flat-sequence {
              frame #0 {
                n196 = call "fgv_NtripClient_stop.vi"("cmd"=cmd_ini-RW."read") -> ("local stops out"=w262:T30)  [unwired: 10 in]
                n197 = Bundle By Name(cluster=w262, "Send serial"=TRUE ("Ntrip tcp")) -> (w261:T30)
                n198 = call "fgv_NtripClient_stop.vi"("cmd"=cmd_ini-RW."write", "local stops"=w261) -> ()  [unwired: 9 in, 1 out]
              }
            }
          }
          frame True {
            n199 = flat-sequence {
              frame #0 {
                n200 = call "fgv_NtripClient_stop.vi"("cmd"=cmd_ini-RW."read") -> ("local stops out"=w267:T30)  [unwired: 10 in]
                n201 = Bundle By Name(cluster=w267, "Send serial"=FALSE ("Ntrip tcp")) -> (w266:T30)
                n202 = call "fgv_NtripClient_stop.vi"("cmd"=cmd_ini-RW."write", "local stops"=w266) -> ()  [unwired: 9 in, 1 out]
              }
              frame #1 {
                n203 = call "fgv_Send-Serial_Q.vi"("cmd"=enum16{"create", "write", "read", "close"}."write", "data"=enum16{"run", "check", "stop"}."run") -> ()  [unwired: 8 in, 2 out]
              }
            }
          }
        }
      }
      event "GNSS Start-Stop": Value Change {
        n204 = event-data() -> ()  [unwired: 1 in, 1 out]
        n205 = case shown="True" "GNSS Start-Stop" {
          frame False {
            n206 = flat-sequence {
              frame #0 {
                n207 = call "fgv_NtripClient_stop.vi"("cmd"=cmd_ini-RW."read") -> ("local stops out"=w275:T30)  [unwired: 10 in]
                n208 = Bundle By Name(cluster=w275, "GNSS serial"=TRUE ("Ntrip tcp")) -> (w274:T30)
                n209 = call "fgv_NtripClient_stop.vi"("cmd"=cmd_ini-RW."write", "local stops"=w274) -> ()  [unwired: 9 in, 1 out]
              }
            }
          }
          frame True {
            n210 = flat-sequence {
              frame #0 {
                n211 = call "fgv_NtripClient_stop.vi"("cmd"=cmd_ini-RW."read") -> ("local stops out"=w280:T30)  [unwired: 10 in]
                n212 = Bundle By Name(cluster=w280, "GNSS serial"=FALSE ("Ntrip tcp")) -> (w279:T30)
                n213 = call "fgv_NtripClient_stop.vi"("cmd"=cmd_ini-RW."write", "local stops"=w279) -> ()  [unwired: 9 in, 1 out]
              }
              frame #1 {
                n214 = call "fgv_GNSS_Serial_Q.vi"("cmd"=enum16{"create", "write", "read", "close"}."write", "data"=enum16{"run", "check", "stop"}."run") -> ()  [unwired: 8 in, 2 out]
              }
            }
          }
        }
      }
      event "Sel NMEA type": Value Change; "Sel NMEA type": Mouse Down {
        n215 = event-data() -> ()  [unwired: 1 in, 1 out]
        n216 = call "fgv_NtripClient_config.vi"("cmd"=cmd_common."read") -> ("config val out"=w289:T19)  [unwired: 10 in]
        n217 = Bundle By Name(cluster=w289, "Sel NMEA type"="Sel NMEA type") -> (w288:T19)
        n218 = call "fgv_NtripClient_config.vi"("cmd"=cmd_common."write", "config val"=w288) -> ()  [unwired: 9 in, 1 out]
      }
      event "Select Mount points": Value Change; "Select Mount points": Mouse Down {
        n219 = event-data() -> ()  [unwired: 1 in, 4 out]
        n220 = property on="Select Mount points" class="Ring (strict)"() -> ("DisabledEnum"=w290:T15)  [unwired: 2 in, 2 out]
        n221 = case shown="\"Enabled\", Default" w290 {
          frame "Enabled", Default {
            n222 = local read "Ntrip accounts DB index"() -> (w296:u32)
            n223 = local read "Ntrip accounts DB"() -> (w297:T10[])
            n224 = property on="Select Mount points" class="Ring (strict)"() -> ("Strings []"=w298:string[])  [unwired: 2 in, 2 out]
            n225 = Index Array(array=w297, index=w296) -> (element=w295:T10)
            n226 = Index Array(array=w298, index="Select Mount points") -> (element=w294:string)
            n227 = Bundle By Name(cluster=w295, "ref pt"=w294) -> (w293:T10)
            n228 = Replace Array Subset(array=w297, new element=w293, index=w296) -> (w292:T10[])
            n229 = disable-structure shown="비활성화" {
              disable-tunnel: "Select Mount points" -> [w299 _]
              frame Disabled {
                n230 = flat-sequence {
                  tunnel: w299 -> [_]
                  frame #0 {
                    n231 = call "fgv_NtripClient_config.vi"("cmd"=cmd_common."read") -> ("config val out"=w303:T19)  [unwired: 10 in]
                    n232 = Bundle By Name(cluster=w303) -> (w302:T19)  [unwired: 1 in]
                    n233 = call "fgv_NtripClient_config.vi"("cmd"=cmd_common."write", "config val"=w302) -> ()  [unwired: 9 in, 1 out]
                  }
                }
              }
              frame Enabled {
              }
            }
            n234 = local write "Ntrip accounts DB"(w292) -> ()
          }
          frame "Disabled" {
          }
          frame "Disabled and Grayed Out" {
          }
        }
      }
      event "Local Time offset": Value Change {
        n235 = event-data() -> ()  [unwired: 1 in, 1 out]
        n236 = call "fgv_NtripClient_config.vi"("cmd"=cmd_common."read") -> ("config val out"=w306:T19)  [unwired: 10 in]
        n237 = Bundle By Name(cluster=w306, "Local Time offset"="Local Time offset") -> (w304:T19)
        n238 = call "fgv_NtripClient_config.vi"("cmd"=cmd_common."write", "config val"=w304) -> ()  [unwired: 9 in, 1 out]
      }
      event "Ntrip accounts DB index": Value Change; "Ntrip accounts DB index": Mouse Down {
        n239 = event-data() -> ()  [unwired: 1 in, 1 out]
        n240 = Build Array("Ntrip accounts DB index") -> (w316:u32[])
        n241 = property on="Ntrip accounts DB" class="Arr (strict)"("Index Values"=w316) -> ()  [unwired: 2 in, 2 out]
        n242 = property on="Select Mount points" class="Ring (strict)"("DisabledEnum"=T15."Disabled and Grayed Out" ("비활성화")) -> ()  [unwired: 2 in, 2 out]
        n243 = call "fgv_NtripClient_config.vi"("cmd"=cmd_common."read") -> ("config val out"=w315:T19)  [unwired: 10 in]
        n244 = Bundle By Name(cluster=w315, "Ntrip accounts DB"="Ntrip accounts DB", "Ntrip account DB index"="Ntrip accounts DB index") -> (w314:T19)
        n245 = call "fgv_NtripClient_config.vi"("cmd"=cmd_common."write", "config val"=w314) -> ()  [unwired: 9 in, 1 out]
      }
      event "GNSS Serial delay": Value Change {
        n246 = event-data() -> ()  [unwired: 1 in, 1 out]
        n247 = call "fgv_NtripClient_config.vi"("cmd"=cmd_common."read") -> ("config val out"=w319:T19)  [unwired: 10 in]
        n248 = Bundle By Name(cluster=w319, "GNSS Serial delay"="GNSS Serial delay") -> (w318:T19)
        n249 = call "fgv_NtripClient_config.vi"("cmd"=cmd_common."write", "config val"=w318) -> ()  [unwired: 9 in, 1 out]
      }
      event "TMarr-size limit": Value Change {
        n250 = event-data() -> ()  [unwired: 1 in, 1 out]
        n251 = local read "TMarr-size limit"() -> (w322:i32)
        n252 = property on="TM\nptn" class="Slide (strict)"("Scale.Marker.Selection End"=w322) -> ()  [unwired: 2 in, 2 out]
        n253 = call "fgv_NtripClient_config.vi"("cmd"=cmd_common."read") -> ("config val out"=w326:T19)  [unwired: 10 in]
        n254 = Bundle By Name(cluster=w326, "TMarr limit"=w322) -> (w325:T19)
        n255 = call "fgv_NtripClient_config.vi"("cmd"=cmd_common."write", "config val"=w325) -> ()  [unwired: 9 in, 1 out]
      }
      event "stop": Value Change {
        n256 = event-data() -> ()  [unwired: 1 in, 1 out]
        n257 = call "fgv_GNSS_Serial_Q.vi"("cmd"=enum16{"create", "write", "read", "close"}."close") -> ()  [unwired: 9 in, 2 out]
        n258 = call "fgv_RTCM_TCP_Q.vi"("cmd"=enum16{"create", "write", "read", "close"}."close") -> ()  [unwired: 9 in, 2 out]
        n259 = call "fgv_Send-Serial_Q.vi"("cmd"=enum16{"create", "write", "read", "close"}."close") -> ()  [unwired: 9 in, 2 out]
        n260 = call "fgv_global-stop.vi"("cmd"=enum16{"init", "stop", "read"}."stop") -> ("val_out"=w330:bool)  [unwired: 10 in]
      }
      event "update mount point": Value Change {
        n261 = event-data() -> ()  [unwired: 1 in, 1 out]
        n262 = flat-sequence {
          frame #0 {
            n263 = property on="Select Mount points" class="Ring (strict)"("DisabledEnum"=T15."Enabled" ("비활성화")) -> ()  [unwired: 2 in, 2 out]
          }
          frame #1 {
            n264 = call "fgv_RTCM_TCP_Q.vi"("cmd"=enum16{"create", "write", "read", "close"}."write", "data"=enum16{"run", "check", "stop"}."check") -> ()  [unwired: 8 in, 2 out]
          }
        }
      }
      event "Ntrip accounts DB": Value Change {
        n265 = event-data() -> ()  [unwired: 1 in, 1 out]
        n266 = local read "Ntrip accounts DB"() -> (w335:T10[])
        n267 = call "fgv_NtripClient_config.vi"("cmd"=cmd_common."read") -> ("config val out"=w339:T19)  [unwired: 10 in]
        n268 = Bundle By Name(cluster=w339, "Ntrip accounts DB"=w335) -> (w338:T19)
        n269 = call "fgv_NtripClient_config.vi"("cmd"=cmd_common."write", "config val"=w338) -> ()  [unwired: 9 in, 1 out]
      }
      event "gmap center": Value Change {
        n270 = event-data() -> ()  [unwired: 1 in, 1 out]
        n271 = call "fgv_gmap_core.vi"("cmd"=gmap_fgv-cmd."zoom n center markers") -> ("error out"=w340:errorcluster)  [unwired: 7 in, 3 out]
        n272 = local read "zoom"() -> (w343:dbl)
        n273 = Number To Decimal String(number=w343) -> (decimal integer string=w342:string)  [unwired: 1 in]
        n274 = call "fgv_gmap_core.vi"(7:"cmd"=gmap_fgv-cmd."zoom" ("cmd"), "error in"=w340, 10:"cmd"=w342) -> ()  [unwired: 5 in, 4 out]
      }
      event "Ntrip connect": Value Change {
        n275 = event-data() -> ()  [unwired: 1 in, 1 out]
        n276 = case shown="True" "Ntrip connect" {
          tunnel: [T15."Enabled" ("비활성화") T15."Disabled and Grayed Out" ("비활성화")] -> w345
          frame False {
            n277 = call "fgv_NtripClient_stop.vi"("cmd"=cmd_ini-RW."read") -> ("local stops out"=w350:T30)  [unwired: 10 in]
            n278 = Bundle By Name(cluster=w350, "Ntrip tcp"=TRUE) -> (w349:T30)
            n279 = call "fgv_NtripClient_stop.vi"("cmd"=cmd_ini-RW."write", "local stops"=w349) -> ()  [unwired: 9 in, 1 out]
          }
          frame True {
            n280 = flat-sequence {
              frame #0 {
                n281 = call "fgv_NtripClient_stop.vi"("cmd"=cmd_ini-RW."read") -> ("local stops out"=w358:T30)  [unwired: 10 in]
                n282 = Bundle By Name(cluster=w358, "Ntrip tcp"=FALSE) -> (w357:T30)
                n283 = call "fgv_NtripClient_stop.vi"("cmd"=cmd_ini-RW."write", "local stops"=w357) -> ()  [unwired: 9 in, 1 out]
              }
              frame #1 {
                n284 = call "fgv_RTCM_TCP_Q.vi"("cmd"=enum16{"create", "write", "read", "close"}."write", "data"=enum16{"run", "check", "stop"}."run") -> ()  [unwired: 8 in, 2 out]
              }
            }
          }
        }
        n285 = property on="Select Mount points" class="Ring (strict)"("DisabledEnum"=w345) -> ()  [unwired: 2 in, 2 out]
        n286 = property on="Ntrip accounts DB" class="Arr (strict)"("DisabledEnum"=w345) -> ()  [unwired: 2 in, 2 out]
        n287 = property on="Ntrip accounts DB index" class="Slide (strict)"("DisabledEnum"=w345) -> ()  [unwired: 2 in, 2 out]
        n288 = property on="update mount point" class="Bool"("DisabledEnum"=w345) -> ()  [unwired: 2 in, 2 out]
      }
      event "tm data reset": Value Change {
        # "TM GPS data array reset"
        n289 = event-data() -> ()  [unwired: 1 in, 1 out]
        n290 = case shown="True" "tm data reset" {
          frame False {
          }
          frame True {
            n291 = call "fgv_TM-arr.vi"("cmd"=cmd_ini-add-read."ini") -> ()  [unwired: 10 in, 1 out]
          }
        }
      }
      event "zoom": Value Change {
        n292 = event-data() -> ()  [unwired: 1 in, 1 out]
        n293 = local read "zoom"() -> (w364:dbl)
        n294 = Number To Decimal String(number=w364) -> (decimal integer string=w363:string)  [unwired: 1 in]
        n295 = call "fgv_gmap_core.vi"(7:"cmd"=gmap_fgv-cmd."zoom" ("cmd"), 10:"cmd"=w363) -> ()  [unwired: 6 in, 4 out]
      }
      event "reset statistics": Value Change {
        n296 = event-data() -> ()  [unwired: 1 in, 1 out]
        n297 = call "fgv_gps-mode_history.vi"("cmd"=cmd_ini-RW."ini") -> ("data out"=w368:T20)  [unwired: 10 in]
        n298 = Unbundle(w368) -> ("NA"=w369:u32, "valid"=w373:u32, "DGPS"=w372:u32, "RTK float"=w371:u32, "RTK fixed"=w370:u32)
        n299 = Build Array(w369, w373, w372, w371, w370) -> (w367:u32[])
        n300 = local write "gnss mode cnt"(w367) -> ()
        n301 = local write "Histogram Graph"(cluster{i32[], dbl[]} {[], []} ("Histogram Graph")) -> ()
      }
      event Value Change {
        n302 = event-data() -> ()  [unwired: 1 in, 1 out]
        n303 = local read "GNSS Serial cfg"() -> (w375:T8)
        n304 = call "fgv_gps_config.vi"("cmd"=enum16{"read", "write"}."write", "GNSS cfg"=w375) -> ()  [unwired: 8 in, 2 out]
      }
    }
  }
  n305 = call "sub_GNSS-Serial.vi"("error in"=w6) -> ("error out"=w2:errorcluster)  [unwired: 10 in]
  n306 = call "sub_Gmap4_GNSS-Ntrip.vi"("error in"=w6) -> ("error out"=w3:errorcluster)  [unwired: 10 in]
  n307 = call "sub_Send-Serial.vi"("error in"=w6) -> ("error out"=w4:errorcluster)  [unwired: 10 in]
  n308 = call "sub_NtripClient_TCP.vi"("error in"=w6) -> ("error out"=w5:errorcluster)  [unwired: 10 in]
  n309 = Merge Errors(w2, w3, w4, w5) -> (w1:errorcluster)
  n310 = flat-sequence {
    tunnel: w7 -> [_]
    tunnel: w1 -> [_]
    frame #0 {
      n311 = stacked-sequence {
        frame #0 {
          n312 = local read "GNSS Serial cfg"() -> (w378:T8)
          n313 = call "fgv_gps_config.vi"("cmd"=enum16{"read", "write"}."write", "GNSS cfg"=w378) -> ()  [unwired: 8 in, 2 out]
        }
        frame #1 {
          n314 = local read "Ntrip accounts DB index"() -> (w379:u32)
          n315 = local read "Send Serial delay ms"() -> (w383:u32)
          n316 = local read "Select Mount points"() -> (w390:u16)
          n317 = local read "Ntrip accounts DB"() -> (w391:T10[])
          n318 = local read "Send-Serial config"() -> (w385:T9)
          n319 = local read "GNSS Serial delay"() -> (w384:u32)
          n320 = local read "Local Time offset"() -> (w382:u32)
          n321 = local read "Mount point arr"() -> (w386:string[])
          n322 = local read "TMarr-size limit"() -> (w388:i32)
          n323 = local read "Sel NMEA type"() -> (w387:T7)
          n324 = local read "Ref R size"() -> (w389:dbl)
          n325 = Bundle(cluster=T19 {"Ntrip accounts DB"=[], "Mount points"=0, "Ref r size"=0.0, "TMarr limit"=0, "Sel NMEA type"=enum."$GPGSV", "Local Time offset"=0, "GNSS Serial delay"=0, "Send Serial delay"=0, "Send Serial config"={"NMEA out port"="", "baud rate"=0}, "Mount point arr"=[], "Ntrip account DB index"=20} ("config val out"), "Ntrip accounts DB"=w391, "Mount points"=w390, "Ref r size"=w389, "TMarr limit"=w388, "Sel NMEA type"=w387, "Local Time offset"=w382, "GNSS Serial delay"=w383, "Send Serial delay"=w384, "Send Serial config"=w385, "Mount point arr"=w386, "Ntrip account DB index"=w379) -> (w380:T19)
          n326 = call "fgv_NtripClient_config.vi"("cmd"=cmd_common."write", "config val"=w380) -> ()  [unwired: 9 in, 1 out]
        }
      }
    }
    frame #1 {
      n327 = local write "stop"(TRUE ("stop")) -> ()
      n328 = call "fgv_GNSS-Ntrip_param_save-load.vi"("ctl"=T13."LastRUN Save") -> ()  [unwired: 9 in, 2 out]
    }
  }
